vi "Athesim control.vi"() -> ()   [LabVIEW 2021]
uses:
  <vilib>/DAQmx/create/channels.llb/DAQmx Create Channel (DO-Digital Output).vi
  <vilib>/Instr/_visa.llb/VISA Configure Serial Port (Instr).vi
  <vilib>/DAQmx/write.llb/DAQmx Write (Analog DBL 1Chan 1Samp).vi
  <vilib>/DAQmx/write.llb/DAQmx Write (Digital Bool 1Line 1Point).vi
  <vilib>/DAQmx/read.llb/DAQmx Read (Digital Bool 1Line 1Point).vi
  <vilib>/measure/NI_MABase.lvlib
  <vilib>/DAQmx/create/channels.llb/DAQmx Create Channel (DI-Digital Input).vi
  <vilib>/DAQmx/write.llb/DAQmx Write (Analog Wfm 1Chan NSamp).vi
  <vilib>/DAQmx/create/channels.llb/DAQmx Create Channel (AO-Voltage-Basic).vi
panel:
  out "?":bool
  in  "Go live":bool
  in  "stop":bool=TRUE
  in  "Go SIM":bool
  in  "MG17Motor":refnum<k7>(container)
  in  "Tab Control":T1(tab)
  in  "acquire 405":bool
  in  "405 Exp":dbl=150.0
  out "Images needed":dbl=108.0
  in  "5 phases":bool
  in  "Exposure time":dbl=100.0
  in  "interval /s":dbl
  in  "Timepoints":u32=12 min=1 max=1000 step=1
  in  "647":bool
  in  "561":bool
  in  "488":bool
  in  "405":bool
  in  "Steps /um":dbl
  in  "z-slices":dbl=1.0
  in  "acquire 640":bool=TRUE
  in  "647 Exp":dbl=150.0
  in  "acquire 561":bool=TRUE
  in  "561 Exp":dbl=80.0
  in  "acquire 488":bool=TRUE
  in  "488 Exp":dbl=150.0
  in  "Live mode":T2(radio)=enum."Mirror 3"
  in  "Delay time":u32=50
  in  "Optosplit":T3(radio)=enum."rolling SIM"
  out "odd/even indicator":bool
  out "Current voltage":dbl=0.95 format="%#_13g"
  in  "Boolean":bool
  in  "Radio Buttons":enum32{"V1", "V2", "V3"}(radio)
  in  "Debug":dbl[](array[numeric])
  in  "647 voltages":dbl[][](array[numeric])=[[0.95, 2.25, 3.5], [0.950655, 2.25185, 3.50055], [0.95131, 2.2537, 3.5011]]
  in  "561 voltages":dbl[][](array[numeric])=[[0.95, 2.2, 3.45], [0.9508, 2.2025, 3.454], [0.9516, 2.205, 3.4548]]
  in  "488 voltages":dbl[][](array[numeric])=[[0.95, 2.25, 3.5], [0.950655, 2.25185, 3.50055], [0.95131, 2.2537, 3.5011]]
  in  "405 voltages":dbl[][](array[numeric])=[[1.0, 0.0, 0.0], [0.0, 0.0, 0.0], [0.0, 0.0, 4.0]]
  out "x+y":i32=4
  in  "647 voltages":dbl[][](array[numeric])=[[0.96, 2.2, 3.5], [0.97, 2.2035, 3.5085], [0.975, 2.2045, 3.5118]]
  in  "561 voltages":dbl[][](array[numeric])=[[0.85, 1.91, 3.2], [0.85065, 1.91064, 3.204], [0.85013, 1.91128, 3.208]]
  in  "488 voltages":dbl[][](array[numeric])=[[0.96, 2.2, 3.5], [0.97, 2.2045, 3.51], [0.975, 2.209, 3.52]]
  in  "405 voltages":dbl[][](array[numeric])=[[1.0, 0.0, 0.0], [0.0, 0.0, 0.0], [0.0, 0.0, 4.0]]
  in  "ASI stage channel":refnum<visa-resource-name>="COM5"
  in  "physical channels":tag="Dev1/ao0"
  in  "expose any":tag="Dev1/port0/line5"
  in  "647 Power":ext(slide)=34.85 scale=0.0..100.0
  in  "405 shutter":tag="Dev1/port0/line8"
  in  "561 shutter":tag="Dev1/port0/line0"
  in  "488 shutter":tag="Dev1/port0/line1"
  in  "Busy in":tag="Dev1/port0/line3"
  in  "Exposure out":tag="Dev1/port0/line2"
  in  "647 channel":refnum<visa-resource-name>="COM4"
  in  "561 power":dbl(slide)=0.15584415584415584 min=0.0 max=1.0 step=0.05 scale=0.0..1.0
  in  "Tab Control 2":T4(tab)
  out "Initialisation error":errorcluster
  out "stage error":errorcluster
  out "Camera/galvo error":errorcluster
  out "Laser error":errorcluster
  out "optosplit stage error":errorcluster
  out "resulting string":string="movrel z=0.000000 \r\n"
  out "resulting string 2":string="movrel z=-0.000000 \r\n"
  in  "short delay":dbl=5.0
  in  "long delay":dbl=55.0
  # "o"
  # "o"
  # "o"
  # "o"
  # "o"
  # "o"
  # "o"
  # "o"
  # "o"
  # "o"
  # "o"
  # "o"
  # "-60"
  # "0"
  # "60"
  # "-60"
  # "0"
  # "60"
  # "-60"
  # "0"
  # "60"
  # "-60"
  # "0"
  # "60"
  # "0"
  # "2p/3"
  # "4p/3"
  # "o"
  # "o"
  # "o"
  # "o"
  # "o"
  # "o"
  # "o"
  # "o"
  # "o"
  # "o"
  # "o"
  # "o"
  # "-60"
  # "0"
  # "60"
  # "-60"
  # "0"
  # "60"
  # "-60"
  # "0"
  # "60"
  # "-60"
  # "0"
  # "60"
  # "0"
  # "3p/5"
  # "5p/5"
  # "7p/5"
  # "9p/5"
  # "Camera lines"
  # "Laser control"
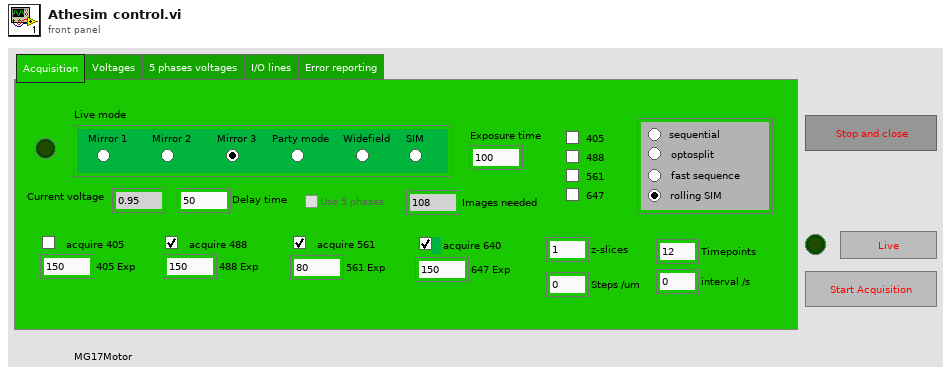
[diagram p1: front panel]
types:
  T1 = enum32{"Acquisition", "Voltages", "5 phases voltages", "I/O lines", "Error reporting"}
  T2 = enum32{"Mirror 1", "Mirror 2", "Mirror 3", "Party mode", "Widefield", "SIM"}
  T3 = enum32{"sequential", "optosplit", "fast sequence", "rolling SIM"}
  T4 = enum32{"Page 1", "Page 2", "Page 3", "Page 4", "Page 5"}
  T5 = enum8{"Enabled", "Disabled", "Disabled and Grayed Out"}
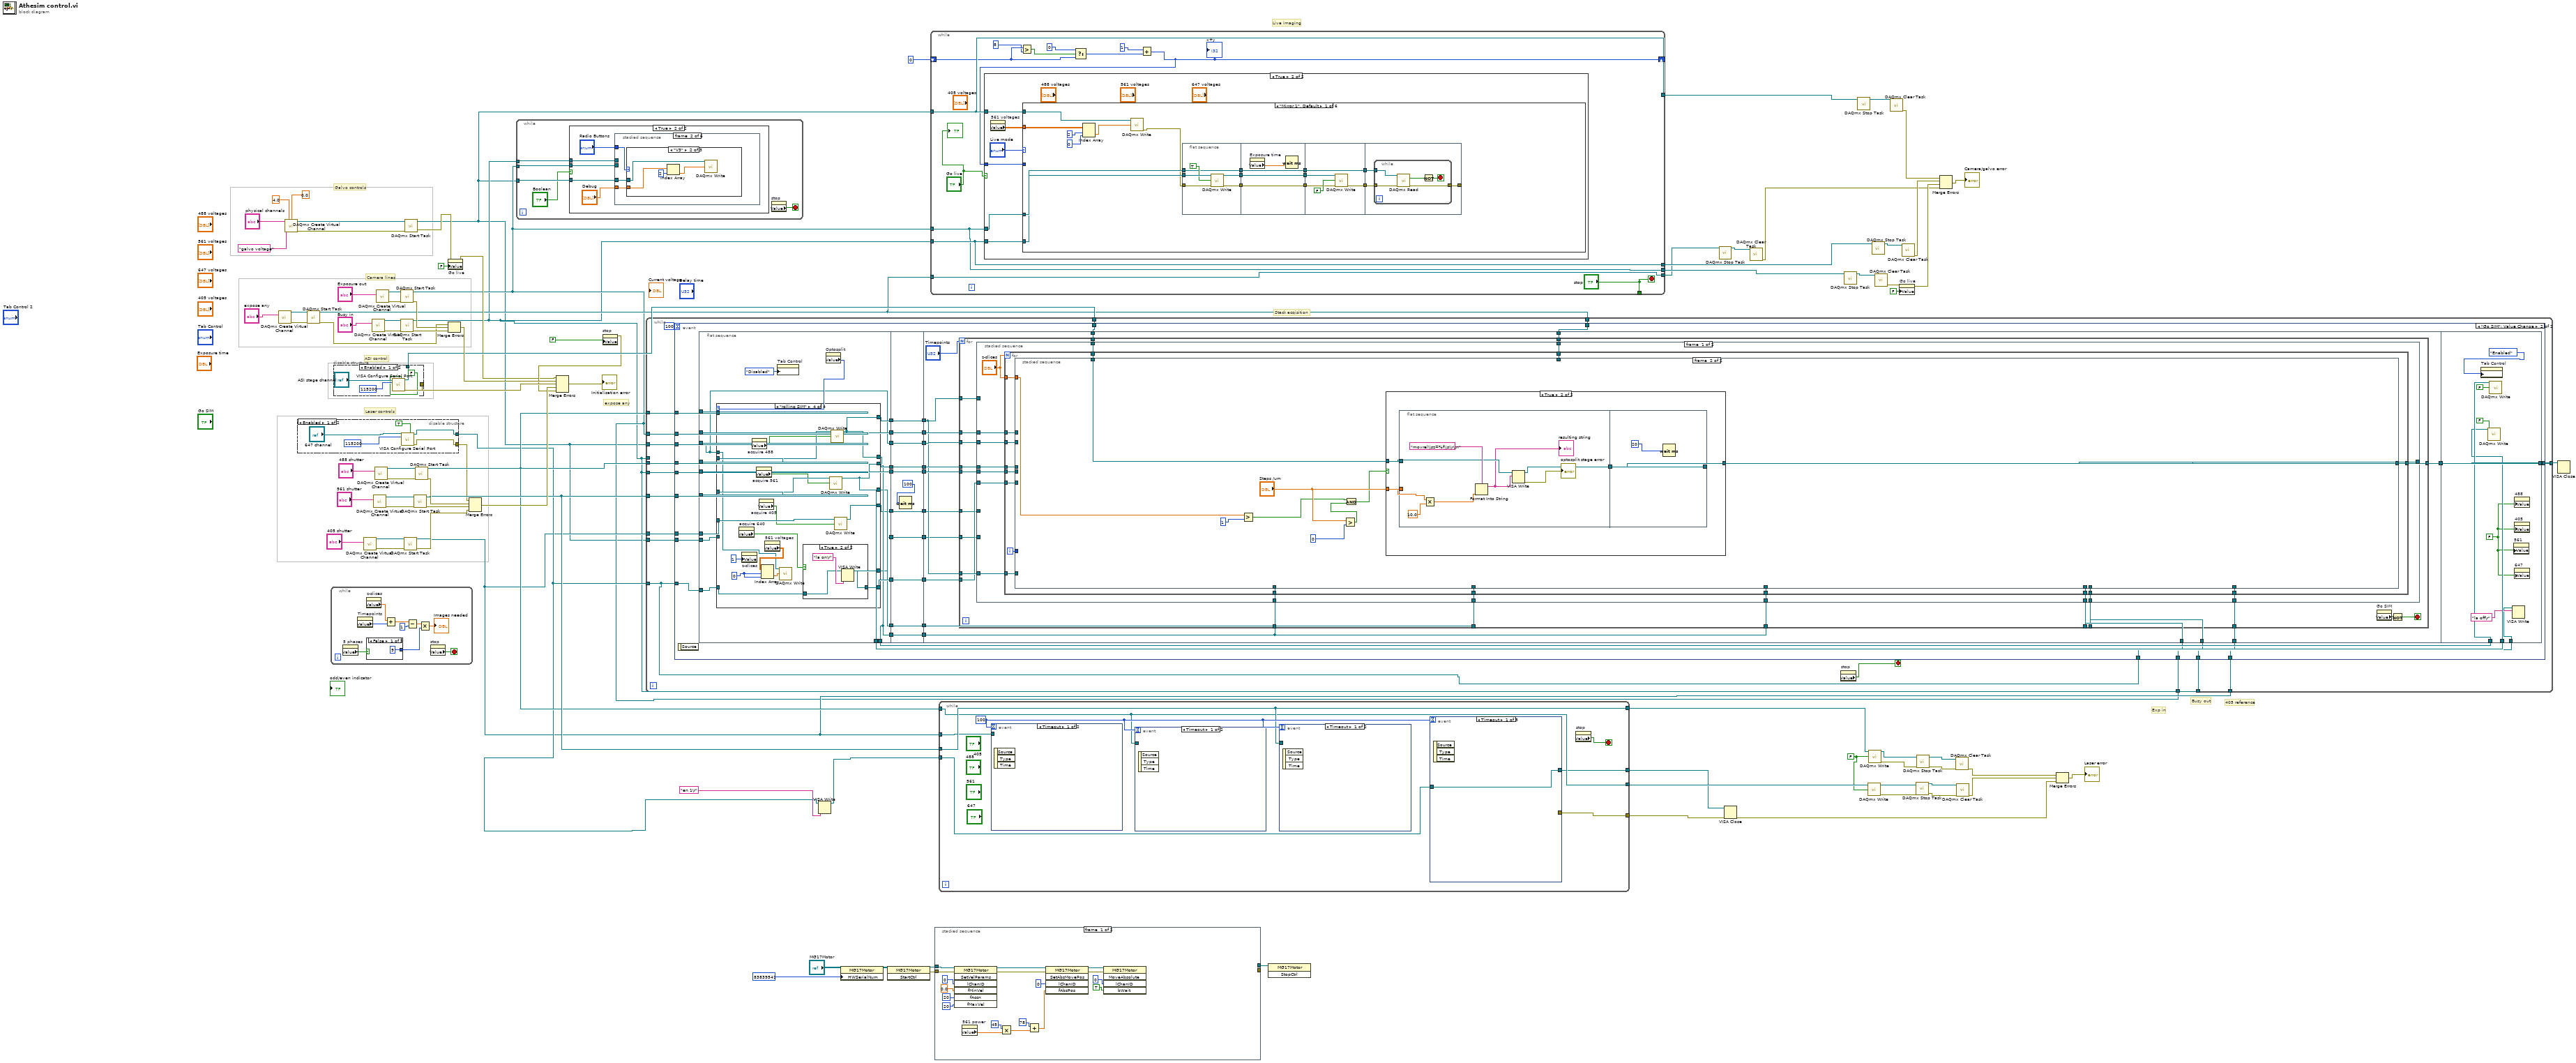
[diagram p0: block diagram]
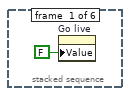
[diagram p3: hidden frame]
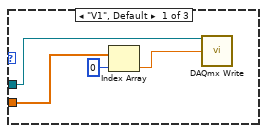
[diagram p4: hidden frame]
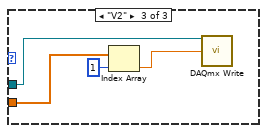
[diagram p5: hidden frame]
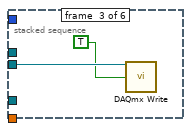
[diagram p6: hidden frame]
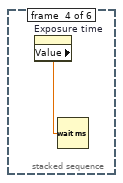
[diagram p7: hidden frame]
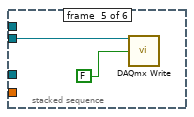
[diagram p8: hidden frame]
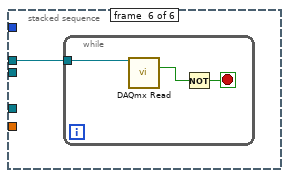
[diagram p9: hidden frame]
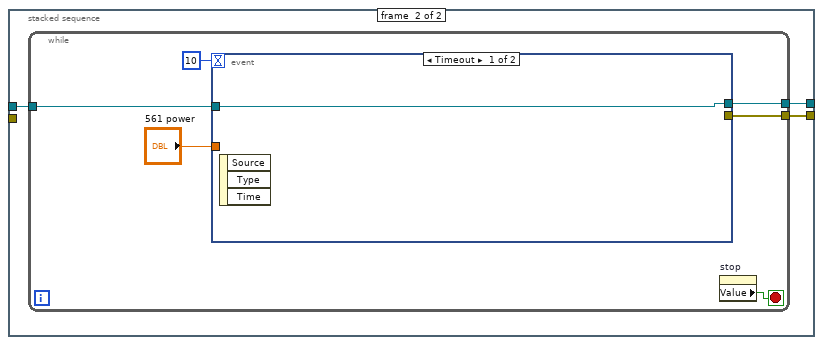
[diagram p10: hidden frame]
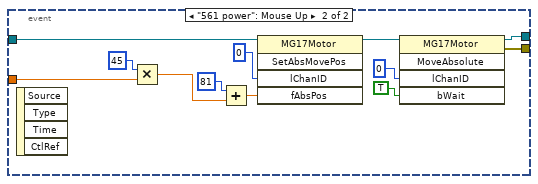
[diagram p11: hidden frame]
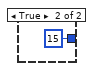
[diagram p13: hidden frame]
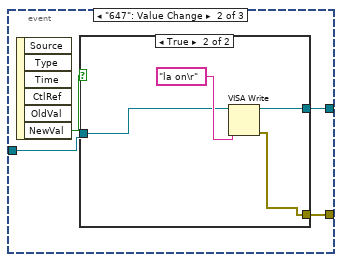
[diagram p15: hidden frame]
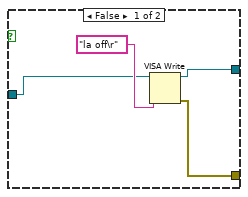
[diagram p16: hidden frame]
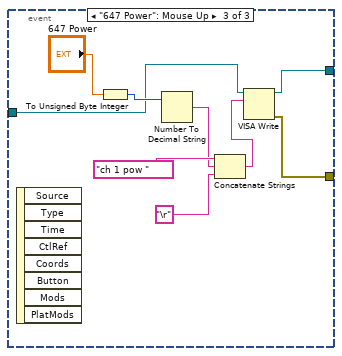
[diagram p17: hidden frame]
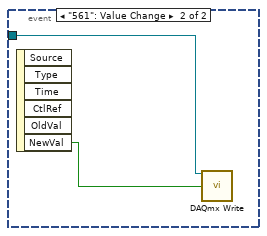
[diagram p18: hidden frame]
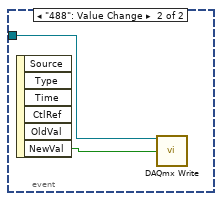
[diagram p19: hidden frame]
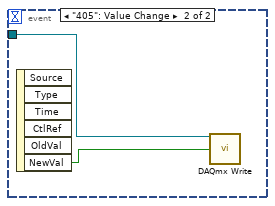
[diagram p20: hidden frame]
diagram:
  w58 = FALSE
  # "expose any"
  # "Busy out"
  # "Exp in"
  # "405 reference"
  # "Stack acqisition"
  # "Live imaging"
  # "Laser controls"
  # "ASI control"
  # "Camera lines"
  # "Galvo controls"
  n1 = call-poly <vilib>:"DAQmx Create Virtual Channel.vi"("lines"="expose any") -> ("task out"=w13:refnum<k21>, "error out"=w12:errorcluster)  [unwired: 13 in]
  n2 = call-poly <vilib>:"DAQmx Create Virtual Channel.vi"("maximum value"=4.0, "minimum value"=0.0, "physical channels"="physical channels", "name to assign"="galvo voltage") -> ("task out"=w6:refnum<k21>, "error out"=w5:errorcluster)  [unwired: 10 in]
  n3 = disable-structure shown="Enabled" {
    disable-tunnel: [w93 _] -> w27
    disable-tunnel: [w92 _] -> w29
    frame Enabled {
      n4 = call-poly "VISA Configure Serial Port"("VISA resource name"="647 channel", "Enable Termination\nChar (T)"=TRUE ("Enable Termination\nChar (T)"), "baud rate (9600)"=u32 115200) -> ("VISA resource name out"=w93:refnum<visa-resource-name>, "error out"=w92:errorcluster)  [unwired: 11 in]
    }
    frame Disabled {
    }
  }
  n5 = call <vilib>:"DAQmx Start Task.vi"("task/channels in"=w13, "error in"=w12) -> ("task out"=w10:refnum<k21>, "error out"=w11:errorcluster)  [unwired: 12 in]
  n6 = while {
    stop <- w97 stop-if-true
    n7 = property on="5 phases" class="Bool (strict)"() -> ("Value"=w105:bool)  [unwired: 2 in, 2 out]
    n8 = property on="Timepoints" class="DigNum (strict)"() -> ("Value"=w101:u32)  [unwired: 2 in, 2 out]
    n9 = property on="z-slices" class="DigNum (strict)"() -> ("Value"=w102:dbl)  [unwired: 2 in, 2 out]
    n10 = case shown="False" w105 {
      tunnel: [9 15] -> w104
      frame False {
      }
      frame True {
      }
    }
    n11 = Add(x=w102, y=w101) -> (x+y=w99:dbl)
    n12 = Subtract(x=w99, y=1) -> (x-y=w98:dbl)
    n13 = Multiply(x=w98, y=w104) -> (x*y=→"Images needed":dbl)
    n14 = property on="stop" class="Bool (strict)"() -> ("Value"=w97:bool)  [unwired: 2 in, 2 out]
  }
  n15 = disable-structure shown="Enabled" {
    disable-tunnel: [w110 _] -> w75
    disable-tunnel: [w109 _] -> w46
    frame Enabled {
      n16 = call-poly "VISA Configure Serial Port"("VISA resource name"="ASI stage channel", "Enable Termination\nChar (T)"=FALSE, "baud rate (9600)"=u32 115200) -> ("VISA resource name out"=w109:refnum<visa-resource-name>, "error out"=w110:errorcluster)  [unwired: 11 in]
    }
    frame Disabled {
    }
  }
  n17 = call-poly <vilib>:"DAQmx Create Virtual Channel.vi"("lines"="405 shutter") -> ("task out"=w40:refnum<k21>, "error out"=w41:errorcluster)  [unwired: 13 in]
  n18 = call-poly <vilib>:"DAQmx Create Virtual Channel.vi"("lines"="Busy in") -> ("task out"=w88:refnum<k21>, "error out"=w89:errorcluster)  [unwired: 13 in]
  n19 = call-poly <vilib>:"DAQmx Create Virtual Channel.vi"("lines"="561 shutter") -> ("task out"=w84:refnum<k21>, "error out"=w85:errorcluster)  [unwired: 13 in]
  n20 = call-poly <vilib>:"DAQmx Create Virtual Channel.vi"("lines"="488 shutter") -> ("task out"=w86:refnum<k21>, "error out"=w87:errorcluster)  [unwired: 13 in]
  n21 = call-poly <vilib>:"DAQmx Create Virtual Channel.vi"("lines"="Exposure out") -> ("task out"=w91:refnum<k21>, "error out"=w90:errorcluster)  [unwired: 13 in]
  n22 = call <vilib>:"DAQmx Start Task.vi"("task/channels in"=w91, "error in"=w90) -> ("task out"=w3:refnum<k21>, "error out"=w77:errorcluster)  [unwired: 12 in]
  n23 = call <vilib>:"DAQmx Start Task.vi"("task/channels in"=w88, "error in"=w89) -> ("task out"=w2:refnum<k21>, "error out"=w76:errorcluster)  [unwired: 12 in]
  n24 = call <vilib>:"DAQmx Start Task.vi"("task/channels in"=w40, "error in"=w41) -> ("task out"=w25:refnum<k21>, "error out"=w39:errorcluster)  [unwired: 12 in]
  n25 = call <vilib>:"DAQmx Start Task.vi"("task/channels in"=w6, "error in"=w5) -> ("task out"=w1:refnum<k21>, "error out"=w23:errorcluster)  [unwired: 12 in]
  n26 = call <vilib>:"DAQmx Start Task.vi"("task/channels in"=w84, "error in"=w85) -> ("task out"=w71:refnum<k21>, "error out"=w78:errorcluster)  [unwired: 12 in]
  n27 = call <vilib>:"DAQmx Start Task.vi"("task/channels in"=w86, "error in"=w87) -> ("task out"=w70:refnum<k21>, "error out"=w79:errorcluster)  [unwired: 12 in]
  n28 = property on="Go live" class="Bool (strict)"(error in=w23, "Value"=FALSE) -> (error out=w22:errorcluster)  [unwired: 1 in, 1 out]
  n29 = Merge Errors(w11, w77, w76) -> (w74:errorcluster)
  n30 = Merge Errors(w29, w79, w78, w39) -> (w73:errorcluster)
  n31 = while {
    tunnel: w3 -> [w116]
    tunnel: w2 -> [w115]
    tunnel: w1 -> [w114]
    stop <- w117 stop-if-true
    n32 = case shown="True" "Boolean" {
      tunnel: w116 -> [_ w122]
      tunnel: w115 -> [_ w121]
      tunnel: w114 -> [_ w120]
      frame False {
      }
      frame True {
        n33 = stacked-sequence {
          tunnel: w122 -> [_ _ w140 _ w142 _]
          tunnel: w121 -> [_ _ _ _ _ w145]
          tunnel: "Radio Buttons" -> [_ w126 _ _ _ _]
          tunnel: "Debug" -> [_ w125 _ _ _ _]
          tunnel: w120 -> [_ w124 _ _ _ _]
          frame #0 {
            n34 = property on="Go live" class="Bool (strict)"("Value"=FALSE ("Go live")) -> ()  [unwired: 2 in, 2 out]
          }
          frame #1 {
            n35 = case shown="\"V3\"" w126 {
              tunnel: w125 -> [w129 w133 w137]
              tunnel: w124 -> [w130 w134 w138]
              frame "V1", Default {
                n36 = Index Array(array=w129, index=0) -> (element=w128:dbl)
                n37 = call-poly <vilib>:"DAQmx Write.vi"("task/channels in"=w130, "data"=w128) -> ()  [unwired: 11 in, 3 out]
              }
              frame "V3" {
                n38 = Index Array(array=w133, index=2) -> (element=w132:dbl)
                n39 = call-poly <vilib>:"DAQmx Write.vi"("task/channels in"=w134, "data"=w132) -> ()  [unwired: 11 in, 3 out]
              }
              frame "V2" {
                n40 = Index Array(array=w137, index=1) -> (element=w136:dbl)
                n41 = call-poly <vilib>:"DAQmx Write.vi"("task/channels in"=w138, "data"=w136) -> ()  [unwired: 11 in, 3 out]
              }
            }
          }
          frame #2 {
            n42 = call-poly <vilib>:"DAQmx Write.vi"("task/channels in"=w140, "data"=TRUE) -> ()  [unwired: 11 in, 3 out]
          }
          frame #3 {
            n43 = property on="Exposure time" class="DigNum (strict)"() -> ("Value"=w141:dbl)  [unwired: 2 in, 2 out]
            n44 = Wait (ms)(milliseconds to wait=w141) -> ()  [unwired: 1 out]
          }
          frame #4 {
            n45 = call-poly <vilib>:"DAQmx Write.vi"("task/channels in"=w142, "data"=FALSE) -> ("error out"=w143:errorcluster)  [unwired: 11 in, 2 out]
          }
          frame #5 {
            n46 = while {
              tunnel: w145 -> [w146]
              stop <- w148 stop-if-true
              n47 = call-poly <vilib>:"DAQmx Read.vi"("task/channels in"=w146) -> ("data"=w147:bool)  [unwired: 12 in, 2 out]
              n48 = Not(x=w147) -> (.not. x?=w148:bool)
            }
          }
        }
      }
    }
    n49 = property on="stop" class="Bool (strict)"() -> ("Value"=w117:bool)  [unwired: 2 in, 2 out]
  }
  n50 = property on="stop" class="Bool (strict)"("Value"=FALSE) -> (error out=w43:errorcluster)  [unwired: 2 in, 1 out]
  n51 = Merge Errors(w22, w74, w75, w73, w43) -> (→"Initialisation error":errorcluster)
  n52 = while {
    tunnel: w3 -> [w164]
    tunnel: w2 -> [w163]
    tunnel: w1 -> [w162]
    tunnel: w70 -> [w161]
    tunnel: w71 -> [w160]
    tunnel: w70 -> [w159]
    tunnel: w46 -> [w157]
    tunnel: [w156] -> w45
    tunnel: w2 -> [_]
    tunnel: w27 -> [w154]
    tunnel: w25 -> [w155]
    tunnel: w25 -> [w153]
    tunnel: w3 -> [w152]
    tunnel: w2 -> [w151]
    tunnel: w1 -> [w150]
    tunnel: w10 -> [w149]
    stop <- w158 stop-if-true
    n53 = event shown="[1] \"Go SIM\": Value Change" {
      selector: _ -> [_ _]
      dyn-events: _ -> [_ _]
      timeout: 100 -> [_ _]
      tunnel: w164 -> [_ w205]
      tunnel: w163 -> [_ w204]
      tunnel: w162 -> [_ w203]
      tunnel: w161 -> [_ w202]
      tunnel: w160 -> [_ w201]
      tunnel: w159 -> [_ w200]
      tunnel: w157 -> [w166 w199]
      tunnel: [w166 w198] -> w156
      tunnel: w154 -> [_ w194]
      tunnel: w155 -> [_ w193]
      tunnel: w154 -> [_ w192]
      tunnel: w153 -> [_ w191]
      tunnel: w152 -> [_ w190]
      tunnel: w151 -> [_ w189]
      tunnel: w150 -> [_ w188]
      tunnel: w149 -> [_ w167]
      event Timeout {
        n54 = event-data() -> ()  [unwired: 1 in, 3 out]
      }
      event "Go SIM": Value Change {
        n55 = event-data() -> ()  [unwired: 1 in, 1 out]
        n56 = flat-sequence {
          tunnel: [w223] -> w187
          tunnel: w205 -> [w223]
          tunnel: [w222] -> w185
          tunnel: w204 -> [w222]
          tunnel: [w207] -> w183
          tunnel: w203 -> [w207]
          tunnel: w202 -> [w220]
          tunnel: w201 -> [w219]
          tunnel: w200 -> [w218]
          tunnel: [w217] -> w181
          tunnel: [w216] -> w179
          tunnel: [w212] -> w195
          tunnel: [w211] -> w196
          tunnel: w194 -> [w215]
          tunnel: w193 -> [w214]
          tunnel: [w213] -> w177
          tunnel: [w212] -> w175
          tunnel: [w211] -> w173
          tunnel: w188 -> [w210]
          tunnel: [w209] -> w170
          tunnel: [w208] -> w168
          tunnel: w187 -> [w313]
          tunnel: [w313] -> w186
          tunnel: w185 -> [w312]
          tunnel: [w312] -> w184
          tunnel: w183 -> [w311]
          tunnel: [w311] -> w182
          tunnel: w181 -> [w310]
          tunnel: [w310] -> w180
          tunnel: w179 -> [w309]
          tunnel: [w309] -> w178
          tunnel: w177 -> [w308]
          tunnel: [w308] -> w176
          tunnel: w175 -> [w307]
          tunnel: [w307] -> w174
          tunnel: w173 -> [w306]
          tunnel: [w306] -> w172
          tunnel: [w304] -> w171
          tunnel: w170 -> [w304]
          tunnel: [w303] -> w169
          tunnel: w168 -> [w303]
          tunnel: w186 -> [w329]
          tunnel: w184 -> [w328]
          tunnel: w182 -> [w327]
          tunnel: w180 -> [w326]
          tunnel: w178 -> [w317]
          tunnel: w199 -> [w325]
          tunnel: [w324] -> w197
          tunnel: w176 -> [w323]
          tunnel: w174 -> [w321]
          tunnel: w172 -> [w322]
          tunnel: w191 -> [w320]
          tunnel: w190 -> [w319]
          tunnel: w189 -> [w318]
          tunnel: w171 -> [w316]
          tunnel: w169 -> [w315]
          tunnel: w167 -> [w314]
          tunnel: [w1125] -> w198
          tunnel: w197 -> [w1125]
          tunnel: w196 -> [w1121]
          tunnel: w195 -> [w1122]
          tunnel: w192 -> [w1119]
          frame #0 {
            n57 = property on="Tab Control" class="TabCtl (strict)"("DisabledEnum"=T5."Disabled" ("Disabled")) -> ()  [unwired: 2 in, 2 out]
            n58 = property on="Optosplit" class="RadioBtnsControl (strict)"() -> ("Value"=w221:T3)  [unwired: 2 in, 2 out]
            n59 = case shown="\"rolling SIM\"" w221 {
              tunnel: w220 -> [_ _ _ _]
              tunnel: w219 -> [w234 w256 w275 w294]
              tunnel: w218 -> [w235 w257 w277 w296]
              tunnel: [w233 w255 w274 w293] -> w217
              tunnel: [w232 w254 w276 w295] -> w216
              tunnel: [w233 w255 w274 w293] -> w211
              tunnel: [w232 w254 w276 w295] -> w212
              tunnel: w215 -> [w227 w249 w272 w292]
              tunnel: w214 -> [w230 w252 w270 w291]
              tunnel: [w224 w246 w268 w289] -> w213
              tunnel: [w228 w250 w269 w290] -> w209
              tunnel: w210 -> [w225 w248 _ _]
              tunnel: [w224 w246 w268 w289] -> w208
              tunnel: w207 -> [_ _ _ w280]
              frame "sequential", Default {
                n60 = property on="odd/even indicator" class="Bool (strict)"() -> ("Value"=w226:bool)  [unwired: 2 in, 2 out]
                n61 = case shown="True" w226 {
                  tunnel: w225 -> [w241 w245]
                  frame False {
                    w239 = 2
                    n62 = property on="647 voltages" class="Arr (strict)"() -> ("Value"=w240:dbl[][])  [unwired: 2 in, 2 out]
                    n63 = Index Array(array=w240, index (row)=w239, index (col)=w239) -> (element=w238:dbl)
                    n64 = call-poly <vilib>:"DAQmx Write.vi"("task/channels in"=w241, "data"=w238) -> ()  [unwired: 11 in, 3 out]
                  }
                  frame True {
                    w243 = 0
                    n65 = property on="561 voltages" class="Arr (strict)"() -> ("Value"=w244:dbl[][])  [unwired: 2 in, 2 out]
                    n66 = Index Array(array=w244, index (row)=w243, index (col)=w243) -> (element=w242:dbl)
                    n67 = call-poly <vilib>:"DAQmx Write.vi"("task/channels in"=w245, "data"=w242) -> ()  [unwired: 11 in, 3 out]
                  }
                }
                n68 = call-poly <vilib>:"DAQmx Write.vi"("task/channels in"=w230, "data"=FALSE) -> ("task out"=w228:refnum<k21>)  [unwired: 11 in, 2 out]
                n69 = call-poly <vilib>:"DAQmx Write.vi"("task/channels in"=w234, "data"=FALSE) -> ("task out"=w233:refnum<k21>)  [unwired: 11 in, 2 out]
                n70 = call-poly <vilib>:"DAQmx Write.vi"("task/channels in"=w235, "data"=FALSE) -> ("task out"=w232:refnum<k21>)  [unwired: 11 in, 2 out]
                n71 = VISA Write(VISA resource name=w227, write buffer="la off\r" ("format string")) -> (VISA resource name out=w224:refnum<visa-resource-name>)  [unwired: 1 in, 2 out]
              }
              frame "fast sequence" {
                n72 = property on="odd/even indicator" class="Bool (strict)"() -> ("Value"=w247:bool)  [unwired: 2 in, 2 out]
                n73 = case shown="True" w247 {
                  tunnel: w248 -> [w263 w267]
                  frame False {
                    w261 = 2
                    n74 = property on="647 voltages" class="Arr (strict)"() -> ("Value"=w262:dbl[][])  [unwired: 2 in, 2 out]
                    n75 = Index Array(array=w262, index (row)=w261, index (col)=w261) -> (element=w260:dbl)
                    n76 = call-poly <vilib>:"DAQmx Write.vi"("task/channels in"=w263, "data"=w260) -> ()  [unwired: 11 in, 3 out]
                  }
                  frame True {
                    w265 = 0
                    n77 = property on="647 voltages" class="Arr (strict)"() -> ("Value"=w266:dbl[][])  [unwired: 2 in, 2 out]
                    n78 = Index Array(array=w266, index (row)=w265, index (col)=w265) -> (element=w264:dbl)
                    n79 = call-poly <vilib>:"DAQmx Write.vi"("task/channels in"=w267, "data"=w264) -> ()  [unwired: 11 in, 3 out]
                  }
                }
                n80 = call-poly <vilib>:"DAQmx Write.vi"("task/channels in"=w252, "data"=FALSE) -> ("task out"=w250:refnum<k21>)  [unwired: 11 in, 2 out]
                n81 = call-poly <vilib>:"DAQmx Write.vi"("task/channels in"=w256, "data"=FALSE) -> ("task out"=w255:refnum<k21>)  [unwired: 11 in, 2 out]
                n82 = call-poly <vilib>:"DAQmx Write.vi"("task/channels in"=w257, "data"=FALSE) -> ("task out"=w254:refnum<k21>)  [unwired: 11 in, 2 out]
                n83 = VISA Write(VISA resource name=w249, write buffer="la off\r" ("format string")) -> (VISA resource name out=w246:refnum<visa-resource-name>)  [unwired: 1 in, 2 out]
              }
              frame "optosplit" {
                n84 = call-poly <vilib>:"DAQmx Write.vi"("task/channels in"=w275, "data"=TRUE) -> ("task out"=w274:refnum<k21>)  [unwired: 11 in, 2 out]
                n85 = call-poly <vilib>:"DAQmx Write.vi"("task/channels in"=w277, "data"=TRUE) -> ("task out"=w276:refnum<k21>)  [unwired: 11 in, 2 out]
                n86 = call-poly <vilib>:"DAQmx Write.vi"("task/channels in"=w270, "data"=TRUE) -> ("task out"=w269:refnum<k21>)  [unwired: 11 in, 2 out]
                n87 = VISA Write(VISA resource name=w272, write buffer="la on\r" ("format string")) -> (VISA resource name out=w268:refnum<visa-resource-name>)  [unwired: 1 in, 2 out]
              }
              frame "rolling SIM" {
                w285 = 0
                n88 = property on="acquire 640" class="Bool (strict)"() -> ("Value"=w281:bool)  [unwired: 2 in, 2 out]
                n89 = property on="z-slices" class="DigNum (strict)"("Value"=1) -> ()  [unwired: 2 in, 2 out]
                n90 = property on="acquire 488" class="Bool (strict)"() -> ("Value"=w284:bool)  [unwired: 2 in, 2 out]
                n91 = property on="acquire 561" class="Bool (strict)"() -> ("Value"=w283:bool)  [unwired: 2 in, 2 out]
                n92 = property on="acquire 405" class="Bool (strict)"() -> ("Value"=w282:bool)  [unwired: 2 in, 2 out]
                n93 = property on="561 voltages" class="Arr (strict)"() -> ("Value"=w286:dbl[][])  [unwired: 2 in, 2 out]
                n94 = Index Array(array=w286, index (row)=w285, index (col)=w285) -> (element=w287:dbl)
                n95 = call-poly <vilib>:"DAQmx Write.vi"("task/channels in"=w280, "data"=w287) -> ()  [unwired: 11 in, 3 out]
                n96 = case shown="True" w281 {
                  tunnel: w292 -> [w298 w301]
                  tunnel: [w297 w300] -> w289
                  frame False {
                    n97 = VISA Write(VISA resource name=w298, write buffer="la off\r" ("format string")) -> (VISA resource name out=w297:refnum<visa-resource-name>)  [unwired: 1 in, 2 out]
                  }
                  frame True {
                    n98 = VISA Write(VISA resource name=w301, write buffer="la on\r" ("format string")) -> (VISA resource name out=w300:refnum<visa-resource-name>)  [unwired: 1 in, 2 out]
                  }
                }
                n99 = call-poly <vilib>:"DAQmx Write.vi"("task/channels in"=w294, "data"=w283) -> ("task out"=w293:refnum<k21>)  [unwired: 11 in, 2 out]
                n100 = call-poly <vilib>:"DAQmx Write.vi"("task/channels in"=w296, "data"=w284) -> ("task out"=w295:refnum<k21>)  [unwired: 11 in, 2 out]
                n101 = call-poly <vilib>:"DAQmx Write.vi"("task/channels in"=w291, "data"=w282) -> ("task out"=w290:refnum<k21>)  [unwired: 11 in, 2 out]
              }
            }
          }
          frame #1 {
            n102 = Wait (ms)(milliseconds to wait=100) -> ()  [unwired: 1 out]
          }
          frame #2 {
            n103 = for {
              N: "Timepoints" -> [_]
              tunnel: w329 -> [w350]
              tunnel: w328 -> [w349]
              tunnel: w327 -> [w348]
              tunnel: w326 -> [w347]
              tunnel: w317 -> [w346]
              tunnel: w325 -> [w345]
              tunnel: [w344] -> w324
              tunnel: w323 -> [w343]
              tunnel: w322 -> [w342]
              tunnel: w321 -> [w341]
              tunnel: w321 -> [w340]
              tunnel: w320 -> [w339]
              tunnel: w319 -> [w338]
              tunnel: w318 -> [w337]
              tunnel: w317 -> [w336]
              tunnel: w316 -> [w335]
              tunnel: w315 -> [w334]
              tunnel: w314 -> [w333]
              stop <- w331 stop-if-true
              n104 = stacked-sequence {
                tunnel: w350 -> [w366 _]
                tunnel: w349 -> [w365 _]
                tunnel: w348 -> [w364 _]
                tunnel: w347 -> [w363 w1030]
                tunnel: w346 -> [w362 _]
                tunnel: w345 -> [w361 w1032]
                tunnel: [w360 _] -> w344
                tunnel: w343 -> [w359 _]
                tunnel: w342 -> [w358 _]
                tunnel: w341 -> [w357 _]
                tunnel: w340 -> [w356 _]
                tunnel: w339 -> [w355 _]
                tunnel: w338 -> [w354 _]
                tunnel: w337 -> [w353 _]
                tunnel: w336 -> [_ w1031]
                tunnel: w335 -> [_ w1029]
                tunnel: w334 -> [_ w1028]
                tunnel: w333 -> [w351 _]
                frame #0 {
                  n105 = for {
                    N: "z-slices" -> [_]
                    tunnel: w366 -> [w383]
                    tunnel: w365 -> [w382]
                    tunnel: w364 -> [w381]
                    tunnel: w363 -> [w380]
                    tunnel: w362 -> [w379]
                    tunnel: w361 -> [w378]
                    tunnel: [w377] -> w360
                    tunnel: w359 -> [w376]
                    tunnel: w358 -> [w375]
                    tunnel: w357 -> [w374]
                    tunnel: w356 -> [w373]
                    tunnel: w355 -> [w372]
                    tunnel: w354 -> [w371]
                    tunnel: w353 -> [w370]
                    tunnel: "z-slices" -> [w368]
                    tunnel: w351 -> [w367]
                    i -> [w369]
                    n106 = stacked-sequence {
                      tunnel: w383 -> [w398 _]
                      tunnel: w382 -> [w397 _]
                      tunnel: w381 -> [w396 _]
                      tunnel: w380 -> [w395 _]
                      tunnel: w379 -> [w394 _]
                      tunnel: w378 -> [_ w1000]
                      tunnel: [_ w999] -> w377
                      tunnel: w376 -> [w392 _]
                      tunnel: w375 -> [w391 _]
                      tunnel: w374 -> [w390 _]
                      tunnel: w373 -> [w389 _]
                      tunnel: w372 -> [w388 _]
                      tunnel: w371 -> [w387 _]
                      tunnel: w370 -> [w386 _]
                      tunnel: w369 -> [w385 _]
                      tunnel: w368 -> [_ w995]
                      tunnel: w367 -> [w384 _]
                      frame #0 {
                        n107 = case shown="\"rolling SIM\"" "Optosplit" {
                          tunnel: w398 -> [w421 w744 w873 w970]
                          tunnel: w397 -> [w420 w743 w872 w969]
                          tunnel: w396 -> [w403 w739 w871 w963]
                          tunnel: w395 -> [w410 _ _ _]
                          tunnel: w394 -> [w409 _ _ _]
                          tunnel: "5 phases" -> [_ _ w870 _]
                          tunnel: w392 -> [w408 w738 _ _]
                          tunnel: w391 -> [w407 w737 _ _]
                          tunnel: w390 -> [w406 _ _ _]
                          tunnel: w389 -> [_ w732 _ _]
                          tunnel: w388 -> [w405 w731 _ _]
                          tunnel: w387 -> [w402 _ _ _]
                          tunnel: w386 -> [w401 _ _ _]
                          tunnel: w385 -> [_ _ _ _]
                          tunnel: w384 -> [w400 w730 w869 w964]
                          frame "sequential", Default {
                            # "Without optosplit"
                            n108 = case shown="True" "acquire 640" {
                              tunnel: w421 -> [w649 w659]
                              tunnel: w420 -> [w647 w658]
                              tunnel: w403 -> [w648 w652]
                              tunnel: [w649 w656] -> w416
                              tunnel: [w648 w657] -> w417
                              tunnel: [w647 w655] -> w418
                              tunnel: w408 -> [_ w651]
                              tunnel: w400 -> [_ w650]
                              frame False {
                              }
                              frame True {
                                n109 = property on="647 voltages" class="Arr (strict)"() -> ("Value"=w653:dbl[][])  [unwired: 2 in, 2 out]
                                n110 = stacked-sequence {
                                seq-local: [_ w673 _ _] -> [_ _ w693 _]
                                seq-local: [_ w672 _ _] -> [_ _ w692 _]
                                seq-local: [_ w671 _ _] -> [_ _ w691 _]
                                seq-local: [_ w670 _ _] -> [_ _ w687 _]
                                seq-local: [_ w669 _ _] -> [_ _ w686 _]
                                tunnel: w659 -> [_ w673 _ _]
                                tunnel: w652 -> [_ w672 _ _]
                                tunnel: w658 -> [_ w671 _ _]
                                tunnel: w653 -> [_ w670 _ _]
                                tunnel: "647 Exp" -> [_ w669 _ _]
                                tunnel: [_ _ w690 _] -> w657
                                tunnel: [_ _ w689 _] -> w656
                                tunnel: [_ _ w688 _] -> w655
                                tunnel: w653 -> [_ w668 _ _]
                                tunnel: w652 -> [_ w667 _ _]
                                tunnel: w651 -> [w660 _ _ w727]
                                tunnel: w650 -> [_ _ w684 _]
                                frame #0 {
                                n111 = stacked-sequence {
                                tunnel: w660 -> [w661 _]
                                frame #0 {
                                n112 = VISA Write(VISA resource name=w661, write buffer="la on\r" ("format string")) -> ()  [unwired: 1 in, 3 out]
                                }
                                frame #1 {
                                n113 = Wait (ms)(milliseconds to wait=100) -> ()  [unwired: 1 out]
                                }
                                }
                                }
                                frame #1 {
                                n114 = property on="odd/even indicator" class="Bool (strict)"() -> ("Value"=w664:bool)  [unwired: 2 in, 2 out]
                                n115 = case shown="False" w664 {
                                tunnel: [2 0] -> w666
                                tunnel: [2 0] -> w665
                                frame False {
                                }
                                frame True {
                                }
                                }
                                n116 = flat-sequence {
                                tunnel: [w681] -> _
                                tunnel: w668 -> [w683]
                                tunnel: w667 -> [w681]
                                tunnel: [w682] -> _
                                tunnel: w666 -> [w679]
                                tunnel: w665 -> [w678]
                                frame #0 {
                                n117 = Index Array(array=w683, index (row)=w679, index (col)=w678) -> (element=w680:dbl)
                                n118 = call-poly <vilib>:"DAQmx Write.vi"("task/channels in"=w681, "data"=w680) -> ("task out"=w682:refnum<k21>)  [unwired: 11 in, 2 out]
                                }
                                }
                                }
                                frame #2 {
                                n119 = for {
                                N: 9 -> [_]
                                tunnel: w687 -> [w705]
                                tunnel: w693 -> [w702]
                                tunnel: w692 -> [w703]
                                tunnel: w691 -> [w701]
                                tunnel: w686 -> [w704]
                                tunnel: [w703] -> w690
                                tunnel: [w702] -> w689
                                tunnel: [w701] -> w688
                                tunnel: w684 -> [w694]
                                i -> [w697]
                                n120 = property on="odd/even indicator" class="Bool (strict)"() -> ("Value"=w695:bool)  [unwired: 2 in, 2 out]
                                n121 = case shown="True" w695 {
                                tunnel: [i32[] [1, 0, 2, 1, 0, 2, 1, 0, 0, 0, 1, 2, 3, 4, 0] i32[] [1, 2, 0, 1, 2, 0, 1, 2, 2, 0, 1, 2, 3, 4, 0]] -> w700
                                tunnel: [i32[] [2, 2, 1, 1, 1, 0, 0, 0, 0, 2, 2, 2, 2, 2, 0] i32[] [0, 0, 1, 1, 1, 2, 2, 2, 2, 2, 2, 2, 2, 2, 0]] -> w699
                                frame False {
                                }
                                frame True {
                                }
                                }
                                n122 = Index Array(array=w700, index=w697) -> (element=w698:i32)
                                n123 = flat-sequence {
                                tunnel: w705 -> [w714]
                                tunnel: w704 -> [w718]
                                tunnel: w703 -> [w717]
                                tunnel: w702 -> [w716]
                                tunnel: w701 -> [w715]
                                tunnel: w696 -> [w712]
                                tunnel: w698 -> [w711]
                                tunnel: w694 -> [w710]
                                frame #0 {
                                n124 = Index Array(array=w714, index (row)=w711, index (col)=w712) -> (element=w713:dbl)
                                n125 = call "take image.vi"("Voltage"=w713, "Exposure time"=w718, "expose any"=w710, "Busy out"=w715, "Exp In"=w716, "Galvo"=w717) -> ()  [unwired: 6 in]
                                }
                                frame #1 {
                                n126 = property on="Delay time" class="DigNum (strict)"() -> ("Value"=w719:u32)  [unwired: 2 in, 2 out]
                                n127 = Wait (ms)(milliseconds to wait=w719) -> ()  [unwired: 1 out]
                                }
                                }
                                n128 = Index Array(array=w699, index=w697) -> (element=w696:i32)
                                }
                                }
                                frame #3 {
                                n129 = property on="acquire 488" class="Bool (strict)"() -> ("Value"=w723:bool)  [unwired: 2 in, 2 out]
                                n130 = property on="acquire 405" class="Bool (strict)"() -> ("Value"=w722:bool)  [unwired: 2 in, 2 out]
                                n131 = property on="acquire 561" class="Bool (strict)"() -> ("Value"=w724:bool)  [unwired: 2 in, 2 out]
                                n132 = property on="odd/even indicator" class="Bool (strict)"() -> ("Value"=w725:bool)  [unwired: 2 in, 2 out]
                                n133 = Or(x=w724, y=w723) -> (x .or. y?=w721:bool)
                                n134 = Not(x=w725) -> (.not. x?=w726:bool)
                                n135 = Or(x=w721, y=w722) -> (x .or. y?=w720:bool)
                                n136 = case shown="True" w720 {
                                tunnel: w727 -> [_ w728]
                                frame False {
                                }
                                frame True {
                                n137 = VISA Write(VISA resource name=w728, write buffer="la off\r" ("format string")) -> ()  [unwired: 1 in, 3 out]
                                }
                                }
                                n138 = property on="odd/even indicator" class="Bool (strict)"("Value"=w726) -> ()  [unwired: 2 in, 2 out]
                                }
                                }
                              }
                            }
                            n139 = case shown="True" "acquire 561" {
                              tunnel: w418 -> [w566 w577]
                              tunnel: w417 -> [w567 w578]
                              tunnel: [w565 w575] -> w414
                              tunnel: [w567 w576] -> w413
                              tunnel: [w566 w574] -> w412
                              tunnel: w416 -> [w565 w573]
                              tunnel: w410 -> [_ _]
                              tunnel: w403 -> [_ w570]
                              tunnel: w407 -> [_ w569]
                              tunnel: w400 -> [_ w568]
                              frame False {
                              }
                              frame True {
                                n140 = property on="561 voltages" class="Arr (strict)"() -> ("Value"=w571:dbl[][])  [unwired: 2 in, 2 out]
                                n141 = stacked-sequence {
                                seq-local: [_ w588 _ _] -> [_ _ w610 _]
                                seq-local: [_ w587 _ _] -> [_ _ w609 _]
                                seq-local: [_ w586 _ _] -> [_ _ w605 _]
                                seq-local: [_ w585 _ _] -> [_ _ w603 _]
                                seq-local: [_ w584 _ _] -> [_ _ w602 _]
                                tunnel: w578 -> [_ w588 _ _]
                                tunnel: w577 -> [_ w587 _ _]
                                tunnel: w573 -> [_ w586 _ _]
                                tunnel: w571 -> [_ w585 _ _]
                                tunnel: "561 Exp" -> [_ w584 _ _]
                                tunnel: [_ _ w608 _] -> w576
                                tunnel: [_ _ w607 _] -> w575
                                tunnel: [_ _ w606 _] -> w574
                                tunnel: w571 -> [_ w582 _ _]
                                tunnel: w570 -> [_ w581 _ _]
                                tunnel: w569 -> [w580 _ _ w644]
                                tunnel: w568 -> [_ _ w601 _]
                                frame #0 {
                                n142 = call-poly <vilib>:"DAQmx Write.vi"("task/channels in"=w580, "data"=TRUE) -> ()  [unwired: 11 in, 3 out]
                                }
                                frame #1 {
                                n143 = flat-sequence {
                                tunnel: w582 -> [w592]
                                tunnel: [w591] -> w583
                                tunnel: w581 -> [w590]
                                tunnel: [w600] -> _
                                tunnel: w583 -> [w600]
                                frame #0 {
                                n144 = property on="odd/even indicator" class="Bool (strict)"() -> ("Value"=w589:bool)  [unwired: 2 in, 2 out]
                                n145 = case shown="True" w589 {
                                tunnel: [2 0] -> w595
                                tunnel: [2 0] -> w594
                                frame False {
                                }
                                frame True {
                                }
                                }
                                n146 = Index Array(array=w592, index (row)=w595, index (col)=w594) -> (element=w593:dbl)
                                n147 = call-poly <vilib>:"DAQmx Write.vi"("task/channels in"=w590, "data"=w593) -> ("task out"=w591:refnum<k21>)  [unwired: 11 in, 2 out]
                                }
                                frame #1 {
                                }
                                }
                                }
                                frame #2 {
                                n148 = for {
                                N: 9 -> [_]
                                tunnel: w603 -> [w622]
                                tunnel: w605 -> [w619]
                                tunnel: w610 -> [w620]
                                tunnel: w609 -> [w618]
                                tunnel: w602 -> [w621]
                                tunnel: [w620] -> w608
                                tunnel: [w619] -> w607
                                tunnel: [w618] -> w606
                                tunnel: w601 -> [w611]
                                i -> [w615]
                                n149 = property on="odd/even indicator" class="Bool (strict)"() -> ("Value"=w612:bool)  [unwired: 2 in, 2 out]
                                n150 = case shown="False" w612 {
                                tunnel: [i32[] [2, 2, 1, 1, 1, 0, 0, 0, 0, 2, 2, 2, 2, 2, 0] i32[] [0, 0, 1, 1, 1, 2, 2, 2, 2, 2, 2, 2, 2, 2, 0]] -> w617
                                tunnel: [i32[] [1, 0, 2, 1, 0, 2, 1, 0, 0, 0, 1, 2, 3, 4, 0] i32[] [1, 2, 0, 1, 2, 0, 1, 2, 2, 0, 1, 2, 3, 4, 0]] -> w616
                                frame False {
                                }
                                frame True {
                                }
                                }
                                n151 = flat-sequence {
                                tunnel: w622 -> [w631]
                                tunnel: w621 -> [w635]
                                tunnel: w620 -> [w634]
                                tunnel: w619 -> [w633]
                                tunnel: w618 -> [w632]
                                tunnel: w614 -> [w629]
                                tunnel: w613 -> [w628]
                                tunnel: w611 -> [w627]
                                frame #0 {
                                n152 = Index Array(array=w631, index (row)=w629, index (col)=w628) -> (element=w630:dbl)
                                n153 = call "take image.vi"("Voltage"=w630, "Exposure time"=w635, "expose any"=w627, "Busy out"=w632, "Exp In"=w633, "Galvo"=w634) -> ()  [unwired: 6 in]
                                }
                                frame #1 {
                                n154 = property on="Delay time" class="DigNum (strict)"() -> ("Value"=w636:u32)  [unwired: 2 in, 2 out]
                                n155 = Wait (ms)(milliseconds to wait=w636) -> ()  [unwired: 1 out]
                                }
                                }
                                n156 = Index Array(array=w616, index=w615) -> (element=w614:i32)
                                n157 = Index Array(array=w617, index=w615) -> (element=w613:i32)
                                }
                                }
                                frame #3 {
                                n158 = property on="acquire 488" class="Bool (strict)"() -> ("Value"=w640:bool)  [unwired: 2 in, 2 out]
                                n159 = property on="acquire 405" class="Bool (strict)"() -> ("Value"=w641:bool)  [unwired: 2 in, 2 out]
                                n160 = property on="acquire 640" class="Bool (strict)"() -> ("Value"=w639:bool)  [unwired: 2 in, 2 out]
                                n161 = Or(x=w640, y=w641) -> (x .or. y?=w638:bool)
                                n162 = Or(x=w638, y=w639) -> (x .or. y?=w637:bool)
                                n163 = case shown="False" w637 {
                                tunnel: w644 -> [_ w645]
                                frame False {
                                }
                                frame True {
                                n164 = call-poly <vilib>:"DAQmx Write.vi"("task/channels in"=w645, "data"=FALSE) -> ()  [unwired: 11 in, 3 out]
                                }
                                }
                                n165 = property on="odd/even indicator" class="Bool (strict)"() -> ("Value"=w643:bool)  [unwired: 2 in, 2 out]
                                n166 = Not(x=w643) -> (.not. x?=w642:bool)
                                n167 = property on="odd/even indicator" class="Bool (strict)"("Value"=w642) -> ()  [unwired: 2 in, 2 out]
                                }
                                }
                              }
                            }
                            n168 = case shown="True" "acquire 488" {
                              tunnel: w414 -> [w487 w493]
                              tunnel: w412 -> [w485 w497]
                              tunnel: w413 -> [w486 w498]
                              tunnel: [w487 w495] -> _
                              tunnel: [w486 w496] -> _
                              tunnel: [w485 w494] -> _
                              tunnel: w409 -> [_ _]
                              tunnel: w403 -> [_ w490]
                              tunnel: w406 -> [_ w489]
                              tunnel: w400 -> [_ w488]
                              frame False {
                              }
                              frame True {
                                n169 = property on="488 voltages" class="Arr (strict)"() -> ("Value"=w491:dbl[][])  [unwired: 2 in, 2 out]
                                n170 = stacked-sequence {
                                seq-local: [_ w507 _ _] -> [_ _ w528 _]
                                seq-local: [_ w506 _ _] -> [_ _ w527 _]
                                seq-local: [_ w505 _ _] -> [_ _ w523 _]
                                seq-local: [_ w504 _ _] -> [_ _ w521 _]
                                seq-local: [_ w503 _ _] -> [_ _ w520 _]
                                tunnel: w498 -> [_ w507 _ _]
                                tunnel: w497 -> [_ w506 _ _]
                                tunnel: w493 -> [_ w505 _ _]
                                tunnel: w491 -> [_ w504 _ _]
                                tunnel: "488 Exp" -> [_ w503 _ _]
                                tunnel: [_ _ w526 _] -> w496
                                tunnel: [_ _ w525 _] -> w495
                                tunnel: [_ _ w524 _] -> w494
                                tunnel: w491 -> [_ w502 _ _]
                                tunnel: w490 -> [_ w501 _ _]
                                tunnel: w489 -> [w499 _ _ w562]
                                tunnel: w488 -> [_ _ w519 _]
                                frame #0 {
                                n171 = call-poly <vilib>:"DAQmx Write.vi"("task/channels in"=w499, "data"=TRUE) -> ()  [unwired: 11 in, 3 out]
                                }
                                frame #1 {
                                n172 = flat-sequence {
                                tunnel: w502 -> [w514]
                                tunnel: w501 -> [w512]
                                tunnel: [w513] -> _
                                frame #0 {
                                n173 = property on="odd/even indicator" class="Bool (strict)"() -> ("Value"=w508:bool)  [unwired: 2 in, 2 out]
                                n174 = case shown="False" w508 {
                                tunnel: [2 0] -> w510
                                tunnel: [2 0] -> w509
                                frame False {
                                }
                                frame True {
                                }
                                }
                                n175 = Index Array(array=w514, index (row)=w510, index (col)=w509) -> (element=w511:dbl)
                                n176 = call-poly <vilib>:"DAQmx Write.vi"("task/channels in"=w512, "data"=w511) -> ("task out"=w513:refnum<k21>)  [unwired: 11 in, 2 out]
                                }
                                }
                                }
                                frame #2 {
                                n177 = for {
                                N: 9 -> [_]
                                tunnel: w521 -> [w540]
                                tunnel: w523 -> [w538]
                                tunnel: w528 -> [w539]
                                tunnel: w527 -> [w537]
                                tunnel: [w539] -> w526
                                tunnel: [w538] -> w525
                                tunnel: [w537] -> w524
                                tunnel: w520 -> [w536]
                                tunnel: w519 -> [w529]
                                i -> [w535]
                                n178 = property on="odd/even indicator" class="Bool (strict)"() -> ("Value"=w530:bool)  [unwired: 2 in, 2 out]
                                n179 = case shown="True" w530 {
                                tunnel: [i32[] [2, 2, 1, 1, 1, 0, 0, 0, 0, 2, 2, 2, 2, 2, 0] i32[] [0, 0, 1, 1, 1, 2, 2, 2, 2, 2, 2, 2, 2, 2, 0]] -> w531
                                tunnel: [i32[] [1, 0, 2, 1, 0, 2, 1, 0, 0, 0, 1, 2, 3, 4, 0] i32[] [1, 2, 0, 1, 2, 0, 1, 2, 2, 0, 1, 2, 3, 4, 0]] -> w532
                                frame False {
                                }
                                frame True {
                                }
                                }
                                n180 = Index Array(array=w532, index=w535) -> (element=w534:i32)
                                n181 = Index Array(array=w531, index=w535) -> (element=w533:i32)
                                n182 = flat-sequence {
                                tunnel: w540 -> [w549]
                                tunnel: w536 -> [w553]
                                tunnel: w539 -> [w552]
                                tunnel: w538 -> [w551]
                                tunnel: w537 -> [w550]
                                tunnel: w534 -> [w547]
                                tunnel: w533 -> [w546]
                                tunnel: w529 -> [w545]
                                frame #0 {
                                n183 = Index Array(array=w549, index (row)=w547, index (col)=w546) -> (element=w548:dbl)
                                n184 = call "take image.vi"("Voltage"=w548, "Exposure time"=w553, "expose any"=w545, "Busy out"=w550, "Exp In"=w551, "Galvo"=w552) -> ()  [unwired: 6 in]
                                }
                                frame #1 {
                                n185 = property on="Delay time" class="DigNum (strict)"() -> ("Value"=w554:u32)  [unwired: 2 in, 2 out]
                                n186 = Wait (ms)(milliseconds to wait=w554) -> ()  [unwired: 1 out]
                                }
                                }
                                }
                                }
                                frame #3 {
                                n187 = property on="acquire 561" class="Bool (strict)"() -> ("Value"=w558:bool)  [unwired: 2 in, 2 out]
                                n188 = property on="acquire 405" class="Bool (strict)"() -> ("Value"=w557:bool)  [unwired: 2 in, 2 out]
                                n189 = property on="acquire 640" class="Bool (strict)"() -> ("Value"=w559:bool)  [unwired: 2 in, 2 out]
                                n190 = property on="odd/even indicator" class="Bool (strict)"() -> ("Value"=w560:bool)  [unwired: 2 in, 2 out]
                                n191 = Not(x=w560) -> (.not. x?=w561:bool)
                                n192 = Or(x=w558, y=w557) -> (x .or. y?=w556:bool)
                                n193 = property on="odd/even indicator" class="Bool (strict)"("Value"=w561) -> ()  [unwired: 2 in, 2 out]
                                n194 = Or(x=w556, y=w559) -> (x .or. y?=w555:bool)
                                n195 = case shown="True" w555 {
                                tunnel: w562 -> [_ w563]
                                frame False {
                                }
                                frame True {
                                n196 = call-poly <vilib>:"DAQmx Write.vi"("task/channels in"=w563, "data"=FALSE) -> ()  [unwired: 11 in, 3 out]
                                }
                                }
                                }
                                }
                              }
                            }
                            n197 = case shown="True" "acquire 405" {
                              tunnel: w405 -> [_ w428]
                              tunnel: w403 -> [_ w426]
                              tunnel: w402 -> [_ w424]
                              tunnel: w401 -> [_ w423]
                              tunnel: w400 -> [_ w422]
                              frame False {
                              }
                              frame True {
                                n198 = property on="405 voltages" class="Arr (strict)"() -> ("Value"=w427:dbl[][])  [unwired: 2 in, 2 out]
                                n199 = stacked-sequence {
                                tunnel: w427 -> [_ w432 w447 _]
                                tunnel: w426 -> [_ w431 w446 _]
                                tunnel: [_ _ _ w482] -> _
                                tunnel: w428 -> [w429 _ _ w482]
                                tunnel: "405 Exp" -> [_ _ w445 _]
                                tunnel: w424 -> [_ _ w444 _]
                                tunnel: w423 -> [_ _ w443 _]
                                tunnel: w422 -> [_ _ w442 _]
                                frame #0 {
                                n200 = call-poly <vilib>:"DAQmx Write.vi"("task/channels in"=w429, "data"=TRUE) -> ()  [unwired: 11 in, 3 out]
                                }
                                frame #1 {
                                n201 = flat-sequence {
                                tunnel: w432 -> [w436]
                                tunnel: [w435] -> w433
                                tunnel: w431 -> [w434]
                                tunnel: [w441] -> _
                                tunnel: w433 -> [w441]
                                frame #0 {
                                n202 = Index Array(array=w436, index (row)=0, index (col)=0) -> (element=w437:dbl)
                                n203 = call-poly <vilib>:"DAQmx Write.vi"("task/channels in"=w434, "data"=w437) -> ("task out"=w435:refnum<k21>)  [unwired: 11 in, 2 out]
                                }
                                frame #1 {
                                n204 = Wait (ms)(milliseconds to wait=50) -> ()  [unwired: 1 out]
                                }
                                }
                                }
                                frame #2 {
                                n205 = for {
                                N: 9 -> [_]
                                tunnel: w447 -> [w458]
                                tunnel: w446 -> [w457]
                                tunnel: w445 -> [w456]
                                tunnel: w444 -> [w455]
                                tunnel: w443 -> [w454]
                                tunnel: w442 -> [w449]
                                i -> [w453]
                                n206 = property on="odd/even indicator" class="Bool (strict)"() -> ("Value"=w450:bool)  [unwired: 2 in, 2 out]
                                n207 = case shown="True" w450 {
                                tunnel: [i32[] [2, 2, 1, 1, 1, 0, 0, 0, 0, 2, 2, 2, 2, 2, 0] i32[] [0, 0, 1, 1, 1, 2, 2, 2, 2, 2, 2, 2, 2, 2, 0]] -> w452
                                tunnel: [i32[] [1, 0, 2, 1, 0, 2, 1, 0, 0, 0, 1, 2, 3, 4, 0] i32[] [1, 2, 0, 1, 2, 0, 1, 2, 2, 0, 1, 2, 3, 4, 0]] -> w451
                                frame False {
                                }
                                frame True {
                                }
                                }
                                n208 = flat-sequence {
                                tunnel: w460 -> [w472]
                                tunnel: w459 -> [w471]
                                tunnel: w458 -> [w470]
                                tunnel: w457 -> [w469]
                                tunnel: w456 -> [w468]
                                tunnel: w455 -> [w467]
                                tunnel: w454 -> [w466]
                                tunnel: w449 -> [w465]
                                frame #0 {
                                n209 = Index Array(array=w470, index (row)=w472, index (col)=w471) -> (element=w473:dbl)
                                n210 = call "take image.vi"("Voltage"=w473, "Exposure time"=w468, "expose any"=w465, "Busy out"=w466, "Exp In"=w467, "Galvo"=w469) -> ()  [unwired: 6 in]
                                }
                                frame #1 {
                                n211 = property on="Delay time" class="DigNum (strict)"() -> ("Value"=w474:u32)  [unwired: 2 in, 2 out]
                                n212 = Wait (ms)(milliseconds to wait=w474) -> ()  [unwired: 1 out]
                                }
                                }
                                n213 = Index Array(array=w451, index=w453) -> (element=w460:i32)
                                n214 = Index Array(array=w452, index=w453) -> (element=w459:i32)
                                }
                                }
                                frame #3 {
                                n215 = property on="acquire 561" class="Bool (strict)"() -> ("Value"=w477:bool)  [unwired: 2 in, 2 out]
                                n216 = property on="acquire 488" class="Bool (strict)"() -> ("Value"=w478:bool)  [unwired: 2 in, 2 out]
                                n217 = property on="acquire 640" class="Bool (strict)"() -> ("Value"=w476:bool)  [unwired: 2 in, 2 out]
                                n218 = Or(x=w477, y=w478) -> (x .or. y?=w479:bool)
                                n219 = property on="odd/even indicator" class="Bool (strict)"() -> ("Value"=w481:bool)  [unwired: 2 in, 2 out]
                                n220 = Or(x=w479, y=w476) -> (x .or. y?=w475:bool)
                                n221 = Not(x=w481) -> (.not. x?=w480:bool)
                                n222 = property on="odd/even indicator" class="Bool (strict)"("Value"=w480) -> ()  [unwired: 2 in, 2 out]
                                n223 = case shown="True" w475 {
                                tunnel: w482 -> [_ w483]
                                frame False {
                                }
                                frame True {
                                n224 = call-poly <vilib>:"DAQmx Write.vi"("task/channels in"=w483, "data"=FALSE) -> ()  [unwired: 11 in, 3 out]
                                }
                                }
                                }
                                }
                              }
                            }
                          }
                          frame "fast sequence" {
                            # "561"
                            # "488"
                            # "fast sequence"
                            n225 = property on="647 Exp" class="DigNum (strict)"() -> ("Value"=w733:dbl)  [unwired: 2 in, 2 out]
                            n226 = property on="647 voltages" class="Arr (strict)"() -> ("Value"=w736:dbl[][])  [unwired: 2 in, 2 out]
                            n227 = stacked-sequence {
                              seq-local: [_ w818 _ _] -> [_ _ w836 _]
                              seq-local: [_ w817 _ _] -> [_ _ w835 _]
                              seq-local: [_ w816 _ _] -> [_ _ w834 _]
                              seq-local: [_ w815 _ _] -> [_ _ w830 _]
                              seq-local: [_ w814 _ _] -> [_ _ w829 _]
                              tunnel: w744 -> [_ w818 _ _]
                              tunnel: w739 -> [_ w817 _ _]
                              tunnel: w743 -> [_ w816 _ _]
                              tunnel: w736 -> [_ w815 _ _]
                              tunnel: w733 -> [_ w814 _ _]
                              tunnel: [_ _ w833 _] -> w741
                              tunnel: [_ _ w832 _] -> w740
                              tunnel: [_ _ w831 _] -> w742
                              tunnel: w736 -> [_ w812 _ _]
                              tunnel: w739 -> [_ w811 _ _]
                              tunnel: w738 -> [w809 _ _ w867]
                              tunnel: w732 -> [w807 _ _ w865]
                              tunnel: w730 -> [_ _ w827 _]
                              frame #0 {
                                n228 = VISA Write(VISA resource name=w809, write buffer="la on\r" ("format string")) -> ()  [unwired: 1 in, 3 out]
                                n229 = call-poly <vilib>:"DAQmx Write.vi"("task/channels in"=w807, "data"=TRUE) -> ()  [unwired: 11 in, 3 out]
                              }
                              frame #1 {
                                n230 = flat-sequence {
                                tunnel: [w819] -> _
                                tunnel: w812 -> [w821]
                                tunnel: [w820] -> w813
                                tunnel: w811 -> [w819]
                                tunnel: [w826] -> _
                                tunnel: w813 -> [w826]
                                frame #0 {
                                n231 = Index Array(array=w821, index (row)=0, index (col)=0) -> (element=w822:dbl)
                                n232 = call-poly <vilib>:"DAQmx Write.vi"("task/channels in"=w819, "data"=w822) -> ("task out"=w820:refnum<k21>)  [unwired: 11 in, 2 out]
                                }
                                frame #1 {
                                n233 = Wait (ms)(milliseconds to wait=50) -> ()  [unwired: 1 out]
                                }
                                }
                              }
                              frame #2 {
                                n234 = for {
                                N: 9 -> [_]
                                tunnel: w830 -> [w848]
                                tunnel: w836 -> [w845]
                                tunnel: w835 -> [w846]
                                tunnel: w834 -> [w844]
                                tunnel: w829 -> [w847]
                                tunnel: [w846] -> w833
                                tunnel: [w845] -> w832
                                tunnel: [w844] -> w831
                                tunnel: w827 -> [w837]
                                i -> [w842]
                                n235 = property on="odd/even indicator" class="Bool (strict)"() -> ("Value"=w840:bool)  [unwired: 2 in, 2 out]
                                n236 = case shown="False" w840 {
                                tunnel: [i32[] [2, 2, 1, 1, 1, 0, 0, 0, 0, 2, 2, 2, 2, 2, 0] i32[] [0, 0, 1, 1, 1, 2, 2, 2, 2, 2, 2, 2, 2, 2, 0]] -> w838
                                tunnel: [i32[] [1, 0, 2, 1, 0, 2, 1, 0, 0, 0, 1, 2, 3, 4, 0] i32[] [1, 2, 0, 1, 2, 0, 1, 2, 2, 0, 1, 2, 3, 4, 0]] -> w839
                                frame False {
                                }
                                frame True {
                                }
                                }
                                n237 = Index Array(array=w839, index=w842) -> (element=w843:i32)
                                n238 = flat-sequence {
                                tunnel: w848 -> [w857]
                                tunnel: w847 -> [w861]
                                tunnel: w846 -> [w860]
                                tunnel: w845 -> [w859]
                                tunnel: w844 -> [w858]
                                tunnel: w841 -> [w855]
                                tunnel: w843 -> [w854]
                                tunnel: w837 -> [w853]
                                frame #0 {
                                n239 = Index Array(array=w857, index (row)=w854, index (col)=w855) -> (element=w856:dbl)
                                n240 = call "take image.vi"("Voltage"=w856, "Exposure time"=w861, "expose any"=w853, "Busy out"=w858, "Exp In"=w859, "Galvo"=w860) -> ()  [unwired: 6 in]
                                }
                                frame #1 {
                                n241 = property on="Delay time" class="DigNum (strict)"() -> ("Value"=w862:u32)  [unwired: 2 in, 2 out]
                                n242 = Wait (ms)(milliseconds to wait=w862) -> ()  [unwired: 1 out]
                                }
                                }
                                n243 = Index Array(array=w838, index=w842) -> (element=w841:i32)
                                }
                              }
                              frame #3 {
                                n244 = property on="odd/even indicator" class="Bool (strict)"() -> ("Value"=w863:bool)  [unwired: 2 in, 2 out]
                                n245 = Not(x=w863) -> (.not. x?=w864:bool)
                                n246 = property on="odd/even indicator" class="Bool (strict)"("Value"=w864) -> ()  [unwired: 2 in, 2 out]
                                n247 = VISA Write(VISA resource name=w867, write buffer="la off\r" ("format string")) -> ()  [unwired: 1 in, 3 out]
                                n248 = call-poly <vilib>:"DAQmx Write.vi"("task/channels in"=w865, "data"=FALSE) -> ()  [unwired: 11 in, 3 out]
                              }
                            }
                            n249 = property on="561 voltages" class="Arr (strict)"() -> ("Value"=w735:dbl[][])  [unwired: 2 in, 2 out]
                            n250 = property on="561 Exp" class="DigNum (strict)"() -> ("Value"=w734:dbl)  [unwired: 2 in, 2 out]
                            n251 = stacked-sequence {
                              seq-local: [_ w756 _ _] -> [_ _ w774 _]
                              seq-local: [_ w755 _ _] -> [_ _ w773 _]
                              seq-local: [_ w754 _ _] -> [_ _ w769 _]
                              seq-local: [_ w753 _ _] -> [_ _ w767 _]
                              seq-local: [_ w752 _ _] -> [_ _ w766 _]
                              tunnel: w741 -> [_ w756 _ _]
                              tunnel: w742 -> [_ w755 _ _]
                              tunnel: w740 -> [_ w754 _ _]
                              tunnel: w735 -> [_ w753 _ _]
                              tunnel: w734 -> [_ w752 _ _]
                              tunnel: [_ _ w772 _] -> _
                              tunnel: [_ _ w771 _] -> _
                              tunnel: [_ _ w770 _] -> _
                              tunnel: w735 -> [_ w750 _ _]
                              tunnel: w739 -> [_ w749 _ _]
                              tunnel: w737 -> [w748 _ _ w805]
                              tunnel: w731 -> [w745 _ _ w803]
                              tunnel: w730 -> [_ _ w765 _]
                              frame #0 {
                                n252 = call-poly <vilib>:"DAQmx Write.vi"("task/channels in"=w748, "data"=TRUE) -> ()  [unwired: 11 in, 3 out]
                                n253 = call-poly <vilib>:"DAQmx Write.vi"("task/channels in"=w745, "data"=TRUE) -> ()  [unwired: 11 in, 3 out]
                              }
                              frame #1 {
                                n254 = flat-sequence {
                                tunnel: w750 -> [w759]
                                tunnel: [w758] -> w751
                                tunnel: w749 -> [w757]
                                tunnel: [w764] -> _
                                tunnel: w751 -> [w764]
                                frame #0 {
                                n255 = Index Array(array=w759, index (row)=0, index (col)=0) -> (element=w760:dbl)
                                n256 = call-poly <vilib>:"DAQmx Write.vi"("task/channels in"=w757, "data"=w760) -> ("task out"=w758:refnum<k21>)  [unwired: 11 in, 2 out]
                                }
                                frame #1 {
                                n257 = Wait (ms)(milliseconds to wait=50) -> ()  [unwired: 1 out]
                                }
                                }
                              }
                              frame #2 {
                                n258 = for {
                                N: 9 -> [_]
                                tunnel: w767 -> [w786]
                                tunnel: w769 -> [w783]
                                tunnel: w774 -> [w784]
                                tunnel: w773 -> [w782]
                                tunnel: w766 -> [w785]
                                tunnel: [w784] -> w772
                                tunnel: [w783] -> w771
                                tunnel: [w782] -> w770
                                tunnel: w765 -> [w775]
                                i -> [w781]
                                n259 = property on="odd/even indicator" class="Bool (strict)"() -> ("Value"=w776:bool)  [unwired: 2 in, 2 out]
                                n260 = case shown="True" w776 {
                                tunnel: [i32[] [2, 2, 1, 1, 1, 0, 0, 0, 0, 2, 2, 2, 2, 2, 0] i32[] [0, 0, 1, 1, 1, 2, 2, 2, 2, 2, 2, 2, 2, 2, 0]] -> w777
                                tunnel: [i32[] [1, 0, 2, 1, 0, 2, 1, 0, 0, 0, 1, 2, 3, 4, 0] i32[] [1, 2, 0, 1, 2, 0, 1, 2, 2, 0, 1, 2, 3, 4, 0]] -> w778
                                frame False {
                                }
                                frame True {
                                }
                                }
                                n261 = Index Array(array=w778, index=w781) -> (element=w780:i32)
                                n262 = Index Array(array=w777, index=w781) -> (element=w779:i32)
                                n263 = flat-sequence {
                                tunnel: w786 -> [w795]
                                tunnel: w785 -> [w799]
                                tunnel: w784 -> [w798]
                                tunnel: w783 -> [w797]
                                tunnel: w782 -> [w796]
                                tunnel: w780 -> [w793]
                                tunnel: w779 -> [w792]
                                tunnel: w775 -> [w791]
                                frame #0 {
                                n264 = Index Array(array=w795, index (row)=w793, index (col)=w792) -> (element=w794:dbl)
                                n265 = call "take image.vi"("Voltage"=w794, "Exposure time"=w799, "expose any"=w791, "Busy out"=w796, "Exp In"=w797, "Galvo"=w798) -> ()  [unwired: 6 in]
                                }
                                frame #1 {
                                n266 = property on="Delay time" class="DigNum (strict)"() -> ("Value"=w800:u32)  [unwired: 2 in, 2 out]
                                n267 = Wait (ms)(milliseconds to wait=w800) -> ()  [unwired: 1 out]
                                }
                                }
                                }
                              }
                              frame #3 {
                                n268 = call-poly <vilib>:"DAQmx Write.vi"("task/channels in"=w805, "data"=FALSE) -> ()  [unwired: 11 in, 3 out]
                                n269 = property on="odd/even indicator" class="Bool (strict)"() -> ("Value"=w802:bool)  [unwired: 2 in, 2 out]
                                n270 = call-poly <vilib>:"DAQmx Write.vi"("task/channels in"=w803, "data"=FALSE) -> ()  [unwired: 11 in, 3 out]
                                n271 = Not(x=w802) -> (.not. x?=w801:bool)
                                n272 = property on="odd/even indicator" class="Bool (strict)"("Value"=w801) -> ()  [unwired: 2 in, 2 out]
                              }
                            }
                          }
                          frame "optosplit" {
                            n273 = case shown="False" w870 {
                              tunnel: w873 -> [w879 w916]
                              tunnel: w872 -> [w878 w915]
                              tunnel: w871 -> [w877 w914]
                              tunnel: w869 -> [_ w908]
                              frame True {
                                w874 = 15
                                # "With optosplit"
                                n274 = flat-sequence {
                                tunnel: w877 -> [w883]
                                tunnel: w876 -> [w882]
                                tunnel: [w881] -> w880
                                tunnel: [w890] -> w875
                                tunnel: w880 -> [w890]
                                frame #0 {
                                n275 = Index Array(array=w882, index (row)=0, index (col)=0) -> (element=w884:dbl)
                                n276 = call-poly <vilib>:"DAQmx Write.vi"("task/channels in"=w883, "data"=w884) -> ("task out"=w881:refnum<k21>)  [unwired: 11 in, 2 out]
                                }
                                frame #1 {
                                n277 = property on="Delay time" class="DigNum (strict)"() -> ("Value"=w889:u32)  [unwired: 2 in, 2 out]
                                n278 = Add(x=w889, y=20) -> (x+y=w888:u32)
                                n279 = Wait (ms)(milliseconds to wait=w888) -> ()  [unwired: 1 out]
                                }
                                }
                                n280 = property on="561 voltages" class="Arr (strict)"() -> ("Value"=w876:dbl[][])  [unwired: 2 in, 2 out]
                                n281 = for {
                                N: w874 -> [_]
                                tunnel: w876 -> [w898]
                                tunnel: w879 -> [w901]
                                tunnel: w878 -> [w900]
                                tunnel: w875 -> [w899]
                                tunnel: w874 -> [_]
                                i -> [w894]
                                n282 = property on="Exposure time" class="DigNum (strict)"() -> ("Value"=w897:dbl)  [unwired: 2 in, 2 out]
                                n283 = Index Array(array=i32[] [1, 2, 3, 4, 0, 1, 2, 3, 4, 0, 1, 2, 3, 4, 0], index=w894) -> (element=w892:i32)
                                n284 = Index Array(array=i32[] [0, 0, 0, 0, 1, 1, 1, 1, 1, 2, 2, 2, 2, 2, 0], index=w894) -> (element=w893:i32)
                                n285 = Index Array(array=w898, index (row)=w892, index (col)=w893) -> (element=w891:dbl)
                                n286 = property on="Current voltage" class="DigNum (strict)"("Value"=w891) -> ()  [unwired: 2 in, 2 out]
                                n287 = flat-sequence {
                                tunnel: w901 -> [w906]
                                tunnel: w900 -> [w905]
                                tunnel: w891 -> [w904]
                                tunnel: w899 -> [w903]
                                tunnel: w897 -> [w902]
                                frame #0 {
                                n288 = call "take image.vi"("Voltage"=w904, "Exposure time"=w902, "Busy out"=w905, "Exp In"=w906, "Galvo"=w903) -> ()  [unwired: 7 in]
                                }
                                frame #1 {
                                n289 = property on="Delay time" class="DigNum (strict)"() -> ("Value"=w907:u32)  [unwired: 2 in, 2 out]
                                n290 = Wait (ms)(milliseconds to wait=w907) -> ()  [unwired: 1 out]
                                }
                                }
                                }
                              }
                              frame False {
                                w911 = 9
                                # "With optosplit"
                                n291 = flat-sequence {
                                tunnel: w914 -> [w923]
                                tunnel: w913 -> [w922]
                                tunnel: [w921] -> w917
                                tunnel: [w932] -> w912
                                tunnel: w917 -> [w932]
                                frame #0 {
                                n292 = property on="odd/even indicator" class="Bool (strict)"() -> ("Value"=w920:bool)  [unwired: 2 in, 2 out]
                                n293 = case shown="False" w920 {
                                tunnel: [2 0] -> w919
                                tunnel: [2 0] -> w918
                                frame False {
                                }
                                frame True {
                                }
                                }
                                n294 = Index Array(array=w922, index (row)=w919, index (col)=w918) -> (element=w924:dbl)
                                n295 = call-poly <vilib>:"DAQmx Write.vi"("task/channels in"=w923, "data"=w924) -> ("task out"=w921:refnum<k21>)  [unwired: 11 in, 2 out]
                                }
                                frame #1 {
                                n296 = property on="Delay time" class="DigNum (strict)"() -> ("Value"=w931:u32)  [unwired: 2 in, 2 out]
                                n297 = Add(x=w931, y=20) -> (x+y=w930:u32)
                                n298 = Wait (ms)(milliseconds to wait=w930) -> ()  [unwired: 1 out]
                                }
                                }
                                n299 = property on="561 voltages" class="Arr (strict)"() -> ("Value"=w913:dbl[][])  [unwired: 2 in, 2 out]
                                n300 = for {
                                N: w911 -> [_]
                                tunnel: w913 -> [w942]
                                tunnel: w916 -> [w945]
                                tunnel: w915 -> [w944]
                                tunnel: w912 -> [w943]
                                tunnel: w911 -> [_]
                                tunnel: [w934] -> w909
                                tunnel: w908 -> [w933]
                                i -> [w940]
                                n301 = property on="odd/even indicator" class="Bool (strict)"() -> ("Value"=w934:bool)  [unwired: 2 in, 2 out]
                                n302 = property on="Exposure time" class="DigNum (strict)"() -> ("Value"=w941:dbl)  [unwired: 2 in, 2 out]
                                n303 = case shown="False" w934 {
                                tunnel: [i32[] [2, 2, 1, 1, 1, 0, 0, 0, 0, 2, 2, 2, 2, 2, 0] i32[] [0, 0, 1, 1, 1, 2, 2, 2, 2, 2, 2, 2, 2, 2, 0]] -> w935
                                tunnel: [i32[] [1, 0, 2, 1, 0, 2, 1, 0, 0, 0, 1, 2, 3, 4, 0] i32[] [1, 2, 0, 1, 2, 0, 1, 2, 2, 0, 1, 2, 3, 4, 0]] -> w936
                                frame False {
                                }
                                frame True {
                                }
                                }
                                n304 = Index Array(array=w936, index=w940) -> (element=w938:i32)
                                n305 = Index Array(array=w935, index=w940) -> (element=w939:i32)
                                n306 = Index Array(array=w942, index (row)=w938, index (col)=w939) -> (element=w937:dbl)
                                n307 = property on="Current voltage" class="DigNum (strict)"("Value"=w937) -> ()  [unwired: 2 in, 2 out]
                                n308 = flat-sequence {
                                tunnel: w945 -> [w955]
                                tunnel: w944 -> [w954]
                                tunnel: w937 -> [w953]
                                tunnel: w943 -> [w952]
                                tunnel: w941 -> [w951]
                                tunnel: w933 -> [w950]
                                frame #0 {
                                n309 = call "take image.vi"("Voltage"=w953, "Exposure time"=w951, "expose any"=w950, "Busy out"=w954, "Exp In"=w955, "Galvo"=w952) -> ()  [unwired: 6 in]
                                }
                                frame #1 {
                                n310 = property on="Delay time" class="DigNum (strict)"() -> ("Value"=w956:u32)  [unwired: 2 in, 2 out]
                                n311 = Wait (ms)(milliseconds to wait=w956) -> ()  [unwired: 1 out]
                                }
                                }
                                }
                                n312 = Not(x=w909) -> (.not. x?=w910:bool)
                                n313 = property on="odd/even indicator" class="Bool (strict)"("Value"=w910) -> ()  [unwired: 2 in, 2 out]
                              }
                            }
                          }
                          frame "rolling SIM" {
                            w960 = 0 ("index")
                            # "Rolling SIM"
                            n314 = Build Array("short delay", "short delay", "long delay") -> (w961:dbl[])
                            n315 = Insert Into Array(array=w961, index=w960, new element=w961) -> (w962:dbl[])
                            n316 = Insert Into Array(array=w962, index=w960, new element=w962) -> (w957:dbl[])
                            n317 = property on="561 voltages" class="Arr (strict)"() -> ("Value"=w968:dbl[][])  [unwired: 2 in, 2 out]
                            n318 = for {
                              N: 12 -> [_]
                              tunnel: w968 -> [w973]
                              tunnel: w970 -> [w984]
                              tunnel: w969 -> [w983]
                              tunnel: [w976] -> w965
                              tunnel: w964 -> [w975]
                              tunnel: w963 -> [w974]
                              tunnel: w957 -> [w971] mode=indexing
                              i -> [w972]
                              n319 = property on="Exposure time" class="DigNum (strict)"() -> ("Value"=w982:dbl)  [unwired: 2 in, 2 out]
                              n320 = Index Array(array=i32[] [1, 2, 0, 1, 2, 0, 1, 2, 2, 1, 0, 0, 3, 4, 0], index=w972) -> (element=w980:i32)
                              n321 = Index Array(array=i32[] [0, 0, 1, 1, 1, 2, 2, 2, 1, 1, 1, 0, 2, 2, 0], index=w972) -> (element=w981:i32)
                              n322 = Index Array(array=w973, index (row)=w980, index (col)=w981) -> (element=w979:dbl)
                              n323 = property on="Current voltage" class="DigNum (strict)"("Value"=w979) -> ()  [unwired: 2 in, 2 out]
                              n324 = flat-sequence {
                                tunnel: w984 -> [w990]
                                tunnel: w983 -> [w986]
                                tunnel: w979 -> [w989]
                                tunnel: w982 -> [w988]
                                tunnel: w975 -> [w987]
                                tunnel: w974 -> [w985]
                                tunnel: w971 -> [w991]
                                frame #0 {
                                n325 = call "take image.vi"("Voltage"=w989, "Exposure time"=w988, "expose any"=w987, "Busy out"=w986, "Exp In"=w990, "Galvo"=w985) -> ()  [unwired: 6 in]
                                }
                                frame #1 {
                                n326 = Wait (ms)(milliseconds to wait=w991) -> ()  [unwired: 1 out]
                                }
                              }
                              n327 = property on="odd/even indicator" class="Bool (strict)"() -> ("Value"=w976:bool)  [unwired: 2 in, 2 out]
                            }
                            n328 = Not(x=w965) -> (.not. x?=w966:bool)
                            n329 = property on="odd/even indicator" class="Bool (strict)"("Value"=w966) -> ()  [unwired: 2 in, 2 out]
                          }
                        }
                      }
                      frame #1 {
                        n330 = Greater?(x=w995, y=1) -> (0:w994:bool)
                        n331 = Greater?(x="Steps /um", y=0) -> (0:w993:bool)
                        n332 = And(x=w994, y=w993) -> (x .and. y?=w992:bool)
                        n333 = case shown="True" w992 {
                          tunnel: w1000 -> [w1001 w1004]
                          tunnel: [w1001 w1003] -> w999
                          tunnel: "Steps /um" -> [_ w1002]
                          frame False {
                          }
                          frame True {
                            n334 = flat-sequence {
                              tunnel: w1004 -> [w1012]
                              tunnel: [w1011] -> w1005
                              tunnel: w1002 -> [w1008]
                              tunnel: [w1015] -> w1003
                              tunnel: w1005 -> [w1015]
                              frame #0 {
                                n335 = Multiply(x=w1008, y=10.0) -> (x*y=w1006:dbl)
                                n336 = Format Into String "Format Into String"(format string="movrel\\sz=%f\\s\\r\\n", w1006) -> (resulting string=w1009:string)  [unwired: 2 in, 1 out]
                                "resulting string" <- w1009
                                n337 = VISA Write(VISA resource name=w1012, write buffer=w1009) -> (VISA resource name out=w1011:refnum<visa-resource-name>, error out=→"optosplit stage error":errorcluster)  [unwired: 1 in, 1 out]
                              }
                              frame #1 {
                                n338 = Wait (ms)(milliseconds to wait=20) -> ()  [unwired: 1 out]
                              }
                            }
                          }
                        }
                      }
                    }
                  }
                }
                frame #1 {
                  n339 = flat-sequence {
                    tunnel: w1031 -> [w1041]
                    tunnel: w1030 -> [w1040]
                    tunnel: w1029 -> [w1039]
                    tunnel: w1028 -> [w1038]
                    tunnel: [w1037] -> w1025
                    tunnel: [w1036] -> w1022
                    tunnel: [w1035] -> w1019
                    tunnel: [w1034] -> w1018
                    tunnel: w1032 -> [w1065]
                    tunnel: [w1064] -> w1026
                    tunnel: w1025 -> [w1064]
                    tunnel: [w1063] -> w1023
                    tunnel: w1022 -> [w1063]
                    tunnel: [w1062] -> w1020
                    tunnel: w1019 -> [w1062]
                    tunnel: w1018 -> [w1061]
                    tunnel: [w1061] -> w1016
                    tunnel: [w1079] -> w1027
                    tunnel: w1026 -> [w1079]
                    tunnel: [w1078] -> w1024
                    tunnel: w1023 -> [w1078]
                    tunnel: [w1077] -> w1021
                    tunnel: w1020 -> [w1077]
                    tunnel: [w1076] -> w1017
                    tunnel: w1016 -> [w1076]
                    tunnel: w1027 -> [w1086]
                    tunnel: w1024 -> [w1085]
                    tunnel: w1021 -> [w1084]
                    tunnel: w1017 -> [w1083]
                    frame #0 {
                      n340 = case shown="False" FALSE {
                        tunnel: w1041 -> [w1045 w1053]
                        tunnel: w1040 -> [w1044 w1052]
                        tunnel: w1039 -> [w1043 w1051]
                        tunnel: w1038 -> [w1042 w1050]
                        tunnel: [w1042 w1049] -> w1037
                        tunnel: [w1043 w1048] -> w1036
                        tunnel: [w1044 w1047] -> w1035
                        tunnel: [w1045 w1046] -> w1034
                        frame False {
                        }
                        frame True {
                          n341 = call-poly <vilib>:"DAQmx Write.vi"("task/channels in"=w1052, "data"=FALSE) -> ("task out"=w1047:refnum<k21>)  [unwired: 11 in, 2 out]
                          n342 = call-poly <vilib>:"DAQmx Write.vi"("task/channels in"=w1053, "data"=FALSE) -> ("task out"=w1046:refnum<k21>)  [unwired: 11 in, 2 out]
                          n343 = call-poly <vilib>:"DAQmx Write.vi"("task/channels in"=w1051, "data"=FALSE) -> ("task out"=w1048:refnum<k21>)  [unwired: 11 in, 2 out]
                          n344 = VISA Write(VISA resource name=w1050, write buffer="la off\r" ("format string")) -> (VISA resource name out=w1049:refnum<visa-resource-name>)  [unwired: 1 in, 2 out]
                        }
                      }
                    }
                    frame #1 {
                      n345 = property on="z-slices" class="DigNum (strict)"() -> ("Value"=w1059:dbl)  [unwired: 2 in, 2 out]
                      n346 = property on="Optosplit" class="RadioBtnsControl (strict)" props=["Value"]() -> ()  [unwired: 2 in, 3 out]
                      n347 = Greater?(x=w1059, y=1) -> (0:w1058:bool)
                      n348 = case shown="False" w1058 {
                        tunnel: w1065 -> [_ w1072]
                        frame False {
                        }
                        frame True {
                          n349 = property on="z-slices" class="DigNum (strict)"() -> ("Value"=w1070:dbl)  [unwired: 2 in, 2 out]
                          n350 = property on="Steps /um" class="DigNum (strict)"() -> ("Value"=w1071:dbl)  [unwired: 2 in, 2 out]
                          n351 = Negate(x=w1071) -> (-x=w1069:dbl)
                          n352 = Multiply(x=w1069, y=w1070) -> (x*y=w1068:dbl)
                          n353 = Multiply(x=w1068, y=10.0) -> (x*y=w1066:dbl)
                          n354 = Format Into String "Format Into String"(format string="movrel\\sz=%f\\s\\r\\n", w1066) -> (resulting string=w1074:string)  [unwired: 2 in, 1 out]
                          "resulting string 2" <- w1074
                          n355 = VISA Write(VISA resource name=w1072, write buffer=w1074) -> (error out=→"stage error":errorcluster)  [unwired: 1 in, 2 out]
                        }
                      }
                    }
                    frame #2 {
                      n356 = Multiply(x="interval /s", y=1000.0) -> (x*y=w1082:dbl)
                      n357 = Wait (ms)(milliseconds to wait=w1082) -> ()  [unwired: 1 out]
                    }
                    frame #3 {
                      n358 = property on="Optosplit" class="RadioBtnsControl (strict)"() -> ("Value"=w1087:T3)  [unwired: 2 in, 2 out]
                      n359 = disable-structure shown="Disabled" {
                        disable-tunnel: w1087 -> [w1092 _]
                        disable-tunnel: w1086 -> [w1091 _]
                        disable-tunnel: w1085 -> [w1090 _]
                        disable-tunnel: w1084 -> [w1089 _]
                        disable-tunnel: w1083 -> [w1088 _]
                        frame Disabled {
                          n360 = case shown="\"rolling SIM\"" w1092 {
                            tunnel: w1091 -> [_ w1096 w1104 w1112]
                            tunnel: w1090 -> [_ w1095 w1103 w1111]
                            tunnel: w1089 -> [_ w1094 w1102 w1110]
                            tunnel: w1088 -> [_ w1093 w1101 w1109]
                            frame "sequential", Default {
                            }
                            frame "optosplit" {
                              n361 = call-poly <vilib>:"DAQmx Write.vi"("task/channels in"=w1094, "data"=TRUE) -> ()  [unwired: 11 in, 3 out]
                              n362 = call-poly <vilib>:"DAQmx Write.vi"("task/channels in"=w1093, "data"=TRUE) -> ()  [unwired: 11 in, 3 out]
                              n363 = call-poly <vilib>:"DAQmx Write.vi"("task/channels in"=w1095, "data"=TRUE) -> ()  [unwired: 11 in, 3 out]
                              n364 = VISA Write(VISA resource name=w1096, write buffer="la on\r" ("format string")) -> ()  [unwired: 1 in, 3 out]
                            }
                            frame "rolling SIM" {
                              n365 = call-poly <vilib>:"DAQmx Write.vi"("task/channels in"=w1102, "data"=TRUE) -> ()  [unwired: 11 in, 3 out]
                              n366 = call-poly <vilib>:"DAQmx Write.vi"("task/channels in"=w1101, "data"=TRUE) -> ()  [unwired: 11 in, 3 out]
                              n367 = call-poly <vilib>:"DAQmx Write.vi"("task/channels in"=w1103, "data"=TRUE) -> ()  [unwired: 11 in, 3 out]
                              n368 = VISA Write(VISA resource name=w1104, write buffer="la on\r" ("format string")) -> ()  [unwired: 1 in, 3 out]
                            }
                            frame "fast sequence" {
                              n369 = call-poly <vilib>:"DAQmx Write.vi"("task/channels in"=w1110, "data"=TRUE) -> ()  [unwired: 11 in, 3 out]
                              n370 = call-poly <vilib>:"DAQmx Write.vi"("task/channels in"=w1109, "data"=TRUE) -> ()  [unwired: 11 in, 3 out]
                              n371 = call-poly <vilib>:"DAQmx Write.vi"("task/channels in"=w1111, "data"=TRUE) -> ()  [unwired: 11 in, 3 out]
                              n372 = VISA Write(VISA resource name=w1112, write buffer="la on\r" ("format string")) -> ()  [unwired: 1 in, 3 out]
                            }
                          }
                        }
                        frame Enabled {
                        }
                      }
                    }
                  }
                }
              }
              n373 = property on="Go SIM" class="Bool (strict)"() -> ("Value"=w332:bool)  [unwired: 2 in, 2 out]
              n374 = Not(x=w332) -> (.not. x?=w331:bool)
            }
          }
          frame #3 {
            w1118 = FALSE
            n375 = property on="Tab Control" class="TabCtl (strict)"("DisabledEnum"=T5."Enabled" ("Disabled")) -> ()  [unwired: 2 in, 2 out]
            n376 = call-poly <vilib>:"DAQmx Write.vi"("task/channels in"=w1121, "data"=FALSE) -> ()  [unwired: 11 in, 3 out]
            n377 = call-poly <vilib>:"DAQmx Write.vi"("task/channels in"=w1122, "data"=FALSE) -> ()  [unwired: 11 in, 3 out]
            n378 = VISA Write(VISA resource name=w1119, write buffer="la off\r" ("format string")) -> ()  [unwired: 1 in, 3 out]
            n379 = property on="561" class="Bool (strict)"("Value"=w1118) -> ()  [unwired: 2 in, 2 out]
            n380 = property on="488" class="Bool (strict)"("Value"=w1118) -> ()  [unwired: 2 in, 2 out]
            n381 = property on="405" class="Bool (strict)"("Value"=w1118) -> ()  [unwired: 2 in, 2 out]
            n382 = property on="647" class="Bool (strict)"("Value"=w1118) -> ()  [unwired: 2 in, 2 out]
          }
        }
      }
    }
    n383 = property on="stop" class="Bool (strict)"() -> ("Value"=w158:bool)  [unwired: 2 in, 2 out]
  }
  n384 = VISA Write(VISA resource name=w27, write buffer="en 1\r" ("format string")) -> (VISA resource name out=w26:refnum<visa-resource-name>)  [unwired: 1 in, 2 out]
  n385 = property class="MG17Motor"(reference="MG17Motor", "HWSerialNum"=i64 83839541 ("Numeric 2")) -> (reference out=w34:refnum<k7>)  [unwired: 1 in, 1 out]
  n386 = invoke class="MG17Motor" method="StartCtrl"(reference=w34) -> (reference out=w33:refnum<k7>, error out=w32:errorcluster)  [unwired: 2 in, 1 out]
  n387 = while {
    tunnel: w1 -> [w1136]
    tunnel: w3 -> [w1135]
    tunnel: w2 -> [w1137]
    tunnel: ["stop"] -> _
    tunnel: [w1137] -> w68
    tunnel: [w1136] -> w67
    tunnel: [w1135] -> w69
    shift-right: [w1129] -> _
    shift-left: 0 -> [w1128]
    tunnel: w10 -> [w1126]
    tunnel: [w1126] -> w9
    stop <- "stop" stop-if-true
    n388 = Greater?(x=w1128, y=8) -> (0:w1131:bool)
    n389 = Select(t=0, s=w1131, f=w1128) -> (s? t:f=w1130:i32)
    n390 = Add(x=1, y=w1130) -> (x+y=w1129:i32)
    "x+y" <- w1129
    n391 = case shown="True" "Go live" {
      tunnel: w1137 -> [_ w1144]
      tunnel: w1136 -> [_ w1143]
      tunnel: w1135 -> [_ w1142]
      tunnel: w1129 -> [_ w1139]
      frame False {
      }
      frame True {
        n392 = property on="561 voltages" class="Arr (strict)"() -> ("Value"=w1140:dbl[][])  [unwired: 2 in, 2 out]
        n393 = case shown="\"Mirror 1\", Default" "Live mode" {
          tunnel: w1140 -> [w1159 w1202 w1252 w1298 w1329 w1363]
          tunnel: w1143 -> [w1160 w1199 w1238 w1299 w1323 w1362]
          tunnel: w1142 -> [w1147 w1185 w1240 w1286 _ w1361]
          tunnel: w1144 -> [w1146 w1186 w1239 w1285 _ w1356]
          tunnel: w1139 -> [_ _ w1228 _ _ _]
          frame "Mirror 1", Default {
            n394 = Index Array(array=w1159, index (row)=2, index (col)=0) -> (element=w1158:dbl)
            n395 = call-poly <vilib>:"DAQmx Write.vi"("task/channels in"=w1160, "data"=w1158) -> ("error out"=w1145:errorcluster)  [unwired: 11 in, 2 out]
            n396 = flat-sequence {
              tunnel: w1147 -> [w1166]
              tunnel: [w1164] -> w1155
              tunnel: w1145 -> [w1163]
              tunnel: [w1162] -> w1154
              tunnel: w1146 -> [w1161]
              tunnel: [w1161] -> w1153
              tunnel: w1155 -> [w1170]
              tunnel: [w1170] -> w1152
              tunnel: w1154 -> [w1168]
              tunnel: [w1169] -> w1151
              tunnel: w1153 -> [w1169]
              tunnel: [w1168] -> w1150
              tunnel: w1152 -> [w1175]
              tunnel: [w1173] -> w1149
              tunnel: w1151 -> [w1173]
              tunnel: w1150 -> [w1172]
              tunnel: [w1171] -> w1148
              tunnel: w1149 -> [w1178]
              tunnel: w1148 -> [w1177]
              tunnel: [w1176] -> _
              frame #0 {
                n397 = call-poly <vilib>:"DAQmx Write.vi"("task/channels in"=w1166, "data"=TRUE, "error in"=w1163) -> ("task out"=w1164:refnum<k21>, "error out"=w1162:errorcluster)  [unwired: 10 in, 1 out]
              }
              frame #1 {
                n398 = property on="Exposure time" class="DigNum (strict)"() -> ("Value"=w1167:dbl)  [unwired: 2 in, 2 out]
                n399 = Wait (ms)(milliseconds to wait=w1167) -> ()  [unwired: 1 out]
              }
              frame #2 {
                n400 = call-poly <vilib>:"DAQmx Write.vi"("task/channels in"=w1175, "data"=FALSE, "error in"=w1172) -> ("error out"=w1171:errorcluster)  [unwired: 10 in, 2 out]
              }
              frame #3 {
                n401 = while {
                  tunnel: w1178 -> [w1183]
                  tunnel: w1177 -> [w1182]
                  tunnel: [w1181] -> w1176
                  stop <- w1180 stop-if-true
                  n402 = call-poly <vilib>:"DAQmx Read.vi"("task/channels in"=w1183, "error in"=w1182) -> ("data"=w1179:bool, "error out"=w1181:errorcluster)  [unwired: 11 in, 1 out]
                  n403 = Not(x=w1179) -> (.not. x?=w1180:bool)
                }
              }
            }
          }
          frame "Widefield" {
            n404 = Index Array(array=w1202, index (row)=2, index (col)=1) -> ()  [unwired: 1 out]
            n405 = call <vilib>:"Triangle Waveform.vi"("offset"=1.0, "phase"=0.0, "amplitude"=0.06, "frequency"=0.1) -> ("signal out"=w1195:waveform(dbl))  [unwired: 6 in, 1 out]
            n406 = call-poly <vilib>:"DAQmx Write.vi"("task/channels in"=w1199, "data"=w1195) -> ()  [unwired: 11 in, 3 out]
            n407 = flat-sequence {
              tunnel: w1185 -> [w1207]
              tunnel: [w1205] -> w1194
              tunnel: [w1204] -> w1193
              tunnel: [w1203] -> w1192
              tunnel: w1186 -> [w1203]
              tunnel: w1194 -> [w1211]
              tunnel: [w1211] -> w1191
              tunnel: w1193 -> [w1209]
              tunnel: [w1210] -> w1190
              tunnel: w1192 -> [w1210]
              tunnel: [w1209] -> w1189
              tunnel: w1191 -> [w1216]
              tunnel: [w1214] -> w1188
              tunnel: w1190 -> [w1214]
              tunnel: w1189 -> [w1213]
              tunnel: [w1212] -> w1187
              tunnel: w1188 -> [w1219]
              tunnel: w1187 -> [w1218]
              tunnel: [w1217] -> _
              frame #0 {
                n408 = call-poly <vilib>:"DAQmx Write.vi"("task/channels in"=w1207, "data"=TRUE) -> ("task out"=w1205:refnum<k21>, "error out"=w1204:errorcluster)  [unwired: 11 in, 1 out]
              }
              frame #1 {
                n409 = property on="Exposure time" class="DigNum (strict)"() -> ("Value"=w1208:dbl)  [unwired: 2 in, 2 out]
                n410 = Wait (ms)(milliseconds to wait=w1208) -> ()  [unwired: 1 out]
              }
              frame #2 {
                n411 = call-poly <vilib>:"DAQmx Write.vi"("task/channels in"=w1216, "data"=FALSE, "error in"=w1213) -> ("error out"=w1212:errorcluster)  [unwired: 10 in, 2 out]
              }
              frame #3 {
                n412 = while {
                  tunnel: w1219 -> [w1224]
                  tunnel: w1218 -> [w1223]
                  tunnel: [w1222] -> w1217
                  stop <- w1221 stop-if-true
                  n413 = call-poly <vilib>:"DAQmx Read.vi"("task/channels in"=w1224, "error in"=w1223) -> ("data"=w1220:bool, "error out"=w1222:errorcluster)  [unwired: 11 in, 1 out]
                  n414 = Not(x=w1220) -> (.not. x?=w1221:bool)
                }
              }
            }
          }
          frame "SIM" {
            n415 = Quotient & Remainder(x=w1228, y=9) -> (x-y*floor(x/y)=w1250:i32)  [unwired: 1 out]
            n416 = flat-sequence {
              tunnel: w1239 -> [w1256]
              tunnel: w1240 -> [w1257]
              tunnel: [w1257] -> w1237
              tunnel: [w1253] -> w1235
              tunnel: [w1256] -> w1233
              tunnel: w1238 -> [w1255]
              tunnel: w1227 -> [w1254]
              tunnel: w1237 -> [w1261]
              tunnel: [w1261] -> w1236
              tunnel: w1235 -> [w1260]
              tunnel: [w1260] -> w1234
              tunnel: w1233 -> [w1259]
              tunnel: [w1259] -> w1232
              tunnel: [w1265] -> w1248
              tunnel: [w1263] -> w1247
              tunnel: [w1262] -> w1246
              tunnel: w1236 -> [w1267]
              tunnel: w1234 -> [w1264]
              tunnel: w1232 -> [w1262]
              tunnel: w1248 -> [w1271]
              tunnel: [w1271] -> w1245
              tunnel: w1247 -> [w1269]
              tunnel: [w1270] -> w1244
              tunnel: w1246 -> [w1270]
              tunnel: [w1269] -> w1243
              tunnel: w1245 -> [w1276]
              tunnel: [w1274] -> w1242
              tunnel: w1244 -> [w1274]
              tunnel: w1243 -> [w1273]
              tunnel: [w1272] -> w1241
              tunnel: w1242 -> [w1278]
              tunnel: w1241 -> [w1277]
              frame #0 {
                n417 = call-poly <vilib>:"DAQmx Write.vi"("task/channels in"=w1255, "data"=w1254) -> ("error out"=w1253:errorcluster)  [unwired: 11 in, 2 out]
              }
              frame #1 {
                n418 = property on="Delay time" class="DigNum (strict)"() -> ("Value"=w1258:u32)  [unwired: 2 in, 2 out]
                n419 = Wait (ms)(milliseconds to wait=w1258) -> ()  [unwired: 1 out]
              }
              frame #2 {
                n420 = call-poly <vilib>:"DAQmx Write.vi"("task/channels in"=w1267, "data"=TRUE, "error in"=w1264) -> ("task out"=w1265:refnum<k21>, "error out"=w1263:errorcluster)  [unwired: 10 in, 1 out]
              }
              frame #3 {
                n421 = property on="Exposure time" class="DigNum (strict)"() -> ("Value"=w1268:dbl)  [unwired: 2 in, 2 out]
                n422 = Wait (ms)(milliseconds to wait=w1268) -> ()  [unwired: 1 out]
              }
              frame #4 {
                n423 = call-poly <vilib>:"DAQmx Write.vi"("task/channels in"=w1276, "data"=FALSE, "error in"=w1273) -> ("error out"=w1272:errorcluster)  [unwired: 10 in, 2 out]
              }
              frame #5 {
                n424 = while {
                  tunnel: w1278 -> [w1283]
                  tunnel: w1277 -> [w1282]
                  tunnel: [w1281] -> _
                  stop <- w1280 stop-if-true
                  n425 = call-poly <vilib>:"DAQmx Read.vi"("task/channels in"=w1283, "error in"=w1282) -> ("data"=w1279:bool, "error out"=w1281:errorcluster)  [unwired: 11 in, 1 out]
                  n426 = Not(x=w1279) -> (.not. x?=w1280:bool)
                }
              }
            }
            n427 = Add(x=0, y=w1250) -> (x+y=w1229:i32)
            n428 = Index Array(array=i32[] [1, 2, 0, 1, 2, 0, 1, 2, 0, 0, 1, 2, 3, 4, 0], index=w1229) -> (element=w1225:i32)
            n429 = Index Array(array=i32[] [0, 0, 1, 1, 1, 2, 2, 2, 0, 2, 2, 2, 2, 2, 0], index=w1229) -> (element=w1226:i32)
            n430 = Index Array(array=w1252, index (row)=w1225, index (col)=w1226) -> (element=w1227:dbl)
            n431 = property on="Current voltage" class="DigNum (strict)"("Value"=w1227) -> ()  [unwired: 2 in, 2 out]
          }
          frame "Mirror 3" {
            n432 = Index Array(array=w1298, index (row)=2, index (col)=2) -> (element=w1297:dbl)
            n433 = call-poly <vilib>:"DAQmx Write.vi"("task/channels in"=w1299, "data"=w1297) -> ("error out"=w1284:errorcluster)  [unwired: 11 in, 2 out]
            n434 = flat-sequence {
              tunnel: w1286 -> [w1305]
              tunnel: [w1303] -> w1294
              tunnel: w1284 -> [w1302]
              tunnel: [w1301] -> w1293
              tunnel: w1285 -> [w1300]
              tunnel: [w1300] -> w1292
              tunnel: w1294 -> [w1309]
              tunnel: [w1309] -> w1291
              tunnel: w1293 -> [w1307]
              tunnel: [w1308] -> w1290
              tunnel: w1292 -> [w1308]
              tunnel: [w1307] -> w1289
              tunnel: w1291 -> [w1314]
              tunnel: [w1312] -> w1288
              tunnel: w1290 -> [w1312]
              tunnel: w1289 -> [w1311]
              tunnel: [w1310] -> w1287
              tunnel: w1288 -> [w1317]
              tunnel: w1287 -> [w1316]
              tunnel: [w1315] -> _
              frame #0 {
                n435 = call-poly <vilib>:"DAQmx Write.vi"("task/channels in"=w1305, "data"=TRUE, "error in"=w1302) -> ("task out"=w1303:refnum<k21>, "error out"=w1301:errorcluster)  [unwired: 10 in, 1 out]
              }
              frame #1 {
                n436 = property on="Exposure time" class="DigNum (strict)"() -> ("Value"=w1306:dbl)  [unwired: 2 in, 2 out]
                n437 = Wait (ms)(milliseconds to wait=w1306) -> ()  [unwired: 1 out]
              }
              frame #2 {
                n438 = call-poly <vilib>:"DAQmx Write.vi"("task/channels in"=w1314, "data"=FALSE, "error in"=w1311) -> ("error out"=w1310:errorcluster)  [unwired: 10 in, 2 out]
              }
              frame #3 {
                n439 = while {
                  tunnel: w1317 -> [w1322]
                  tunnel: w1316 -> [w1321]
                  tunnel: [w1320] -> w1315
                  stop <- w1318 stop-if-true
                  n440 = call-poly <vilib>:"DAQmx Read.vi"("task/channels in"=w1322, "error in"=w1321) -> ("data"=w1319:bool, "error out"=w1320:errorcluster)  [unwired: 11 in, 1 out]
                  n441 = Not(x=w1319) -> (.not. x?=w1318:bool)
                }
              }
            }
          }
          frame "Party mode" {
            n442 = flat-sequence {
              tunnel: w1329 -> [w1331]
              tunnel: [w1331] -> w1327
              tunnel: w1323 -> [w1330]
              tunnel: [w1336] -> w1328
              tunnel: w1327 -> [w1336]
              tunnel: w1328 -> [w1338]
              tunnel: [w1338] -> w1326
              tunnel: w1323 -> [w1337]
              tunnel: w1326 -> [w1343]
              tunnel: [w1343] -> w1325
              tunnel: w1325 -> [w1345]
              tunnel: [w1345] -> w1324
              tunnel: w1323 -> [w1344]
              tunnel: [w1350] -> _
              tunnel: w1324 -> [w1350]
              frame #0 {
                n443 = Index Array(array=w1331, index (row)=2, index (col)=0) -> (element=w1332:dbl)
                n444 = call-poly <vilib>:"DAQmx Write.vi"("task/channels in"=w1330, "data"=w1332) -> ()  [unwired: 11 in, 3 out]
              }
              frame #1 {
                n445 = property on="Delay time" class="DigNum (strict)"() -> ("Value"=w1335:u32)  [unwired: 2 in, 2 out]
                n446 = Wait (ms)(milliseconds to wait=w1335) -> ()  [unwired: 1 out]
              }
              frame #2 {
                n447 = Index Array(array=w1338, index (row)=2, index (col)=1) -> (element=w1341:dbl)
                n448 = call-poly <vilib>:"DAQmx Write.vi"("task/channels in"=w1337, "data"=w1341) -> ()  [unwired: 11 in, 3 out]
              }
              frame #3 {
                n449 = property on="Delay time" class="DigNum (strict)"() -> ("Value"=w1342:u32)  [unwired: 2 in, 2 out]
                n450 = Wait (ms)(milliseconds to wait=w1342) -> ()  [unwired: 1 out]
              }
              frame #4 {
                n451 = Index Array(array=w1345, index (row)=2, index (col)=2) -> (element=w1346:dbl)
                n452 = call-poly <vilib>:"DAQmx Write.vi"("task/channels in"=w1344, "data"=w1346) -> ()  [unwired: 11 in, 3 out]
              }
              frame #5 {
                n453 = property on="Delay time" class="DigNum (strict)"() -> ("Value"=w1349:u32)  [unwired: 2 in, 2 out]
                n454 = Wait (ms)(milliseconds to wait=w1349) -> ()  [unwired: 1 out]
              }
            }
          }
          frame "Mirror 2" {
            n455 = Index Array(array=w1363, index (row)=2, index (col)=1) -> (element=w1366:dbl)
            n456 = call-poly <vilib>:"DAQmx Write.vi"("task/channels in"=w1362, "data"=w1366) -> ("error out"=w1358:errorcluster)  [unwired: 11 in, 2 out]
            n457 = flat-sequence {
              tunnel: w1361 -> [w1372]
              tunnel: [w1370] -> w1360
              tunnel: w1358 -> [w1369]
              tunnel: [w1368] -> w1357
              tunnel: w1356 -> [w1367]
              tunnel: [w1367] -> w1353
              tunnel: w1360 -> [w1376]
              tunnel: [w1376] -> w1359
              tunnel: w1357 -> [w1374]
              tunnel: [w1375] -> w1354
              tunnel: w1353 -> [w1375]
              tunnel: [w1374] -> w1352
              tunnel: w1359 -> [w1381]
              tunnel: [w1379] -> w1355
              tunnel: w1354 -> [w1379]
              tunnel: w1352 -> [w1378]
              tunnel: [w1377] -> w1351
              tunnel: w1355 -> [w1384]
              tunnel: w1351 -> [w1383]
              tunnel: [w1382] -> _
              frame #0 {
                n458 = call-poly <vilib>:"DAQmx Write.vi"("task/channels in"=w1372, "data"=TRUE, "error in"=w1369) -> ("task out"=w1370:refnum<k21>, "error out"=w1368:errorcluster)  [unwired: 10 in, 1 out]
              }
              frame #1 {
                n459 = property on="Exposure time" class="DigNum (strict)"() -> ("Value"=w1373:dbl)  [unwired: 2 in, 2 out]
                n460 = Wait (ms)(milliseconds to wait=w1373) -> ()  [unwired: 1 out]
              }
              frame #2 {
                n461 = call-poly <vilib>:"DAQmx Write.vi"("task/channels in"=w1381, "data"=FALSE, "error in"=w1378) -> ("error out"=w1377:errorcluster)  [unwired: 10 in, 2 out]
              }
              frame #3 {
                n462 = while {
                  tunnel: w1384 -> [w1389]
                  tunnel: w1383 -> [w1388]
                  tunnel: [w1387] -> w1382
                  stop <- w1386 stop-if-true
                  n463 = call-poly <vilib>:"DAQmx Read.vi"("task/channels in"=w1389, "error in"=w1388) -> ("data"=w1385:bool, "error out"=w1387:errorcluster)  [unwired: 11 in, 1 out]
                  n464 = Not(x=w1385) -> (.not. x?=w1386:bool)
                }
              }
            }
          }
        }
      }
    }
    "?" <- "Go live"
  }
  n465 = stacked-sequence {
    tunnel: w33 -> [w1392 w1410]
    tunnel: w32 -> [w1391 _]
    tunnel: [_ w1409] -> w31
    tunnel: [_ w1408] -> _
    frame #0 {
      n466 = invoke class="MG17Motor" method="SetVelParams"(reference=w1392, error in=w1391, "lChanID"=0, "fMinVel"=0.0, "fAccn"=20, "fMaxVel"=20) -> (reference out=w1399:refnum<k7>, error out=w1398:errorcluster)  [unwired: 1 in, 5 out]
      n467 = property on="561 power" class="Slide (strict)"() -> ("Value"=w1394:dbl)  [unwired: 2 in, 2 out]
      n468 = Multiply(x=45, y=w1394) -> (x*y=w1395:dbl)
      n469 = Add(x=78, y=w1395) -> (x+y=w1393:dbl)
      n470 = invoke class="MG17Motor" method="SetAbsMovePos"(reference=w1399, error in=w1398, "lChanID"=0, "fAbsPos"=w1393) -> (reference out=w1401:refnum<k7>, error out=w1400:errorcluster)  [unwired: 1 in, 3 out]
      n471 = invoke class="MG17Motor" method="MoveAbsolute"(reference=w1401, error in=w1400, "lChanID"=0, "bWait"=TRUE) -> ()  [unwired: 1 in, 5 out]
    }
    frame #1 {
      n472 = while {
        tunnel: [w1416] -> w1409
        tunnel: w1410 -> [w1413]
        tunnel: [w1412] -> w1408
        stop <- w1411 stop-if-true
        n473 = event shown="[0] Timeout" {
          selector: _ -> [_ _]
          dyn-events: _ -> [_ _]
          timeout: 10 -> [_ _]
          tunnel: w1413 -> [w1417 w1425]
          tunnel: [w1417 w1424] -> w1416
          tunnel: "561 power" -> [_ w1420]
          tunnel: [_ w1427] -> w1412
          event Timeout {
            n474 = event-data() -> ()  [unwired: 1 in, 3 out]
          }
          event "561 power": Mouse Up {
            n475 = event-data() -> ()  [unwired: 1 in, 4 out]
            n476 = Multiply(x=45, y=w1420) -> (x*y=w1421:dbl)
            n477 = Add(x=81 ("561 power offset"), y=w1421) -> (x+y=w1419:dbl)
            n478 = invoke class="MG17Motor" method="SetAbsMovePos"(reference=w1425, "lChanID"=0, "fAbsPos"=w1419) -> (reference out=w1423:refnum<k7>)  [unwired: 2 in, 4 out]
            n479 = invoke class="MG17Motor" method="MoveAbsolute"(reference=w1423, "lChanID"=0, "bWait"=TRUE) -> (reference out=w1424:refnum<k7>, error out=w1427:errorcluster)  [unwired: 2 in, 3 out]
          }
        }
        n480 = property on="stop" class="Bool (strict)"() -> ("Value"=w1411:bool)  [unwired: 2 in, 2 out]
      }
    }
  }
  n481 = while {
    tunnel: w70 -> [w1435]
    tunnel: w71 -> [w1436]
    tunnel: [w1436] -> w60
    tunnel: [w1435] -> w59
    tunnel: w26 -> [w1430]
    tunnel: w25 -> [w1433]
    tunnel: [w1432] -> w38
    tunnel: [w1431] -> w37
    stop <- w1434 stop-if-true
    w1437 = 100
    n482 = event shown="[0] Timeout" {
      selector: _ -> [_ _]
      dyn-events: _ -> [_ _]
      timeout: w1437 -> [_ _]
      tunnel: w1433 -> [_ w1464]
      event Timeout {
        n483 = event-data() -> ()  [unwired: 1 in, 3 out]
      }
      event "405": Value Change {
        n484 = event-data() -> ("NewVal"=w1465:bool)  [unwired: 1 in, 5 out]
        n485 = call-poly <vilib>:"DAQmx Write.vi"("task/channels in"=w1464, "data"=w1465) -> ()  [unwired: 11 in, 3 out]
      }
    }
    n486 = event shown="[0] Timeout" {
      selector: _ -> [_ _]
      dyn-events: _ -> [_ _]
      timeout: w1437 -> [_ _]
      tunnel: w1435 -> [_ w1462]
      event Timeout {
        n487 = event-data() -> ()  [unwired: 1 in, 3 out]
      }
      event "488": Value Change {
        n488 = event-data() -> ("NewVal"=w1463:bool)  [unwired: 1 in, 5 out]
        n489 = call-poly <vilib>:"DAQmx Write.vi"("task/channels in"=w1462, "data"=w1463) -> ()  [unwired: 11 in, 3 out]
      }
    }
    n490 = event shown="[0] Timeout" {
      selector: _ -> [_ _]
      dyn-events: _ -> [_ _]
      timeout: w1437 -> [_ _]
      tunnel: w1436 -> [_ w1460]
      event Timeout {
        n491 = event-data() -> ()  [unwired: 1 in, 3 out]
      }
      event "561": Value Change {
        n492 = event-data() -> ("NewVal"=w1461:bool)  [unwired: 1 in, 5 out]
        n493 = call-poly <vilib>:"DAQmx Write.vi"("task/channels in"=w1460, "data"=w1461) -> ()  [unwired: 11 in, 3 out]
      }
    }
    n494 = event shown="[0] Timeout" {
      selector: _ -> [_ _ _]
      dyn-events: _ -> [_ _ _]
      timeout: w1437 -> [_ _ _]
      tunnel: w1430 -> [w1438 w1441 w1455]
      tunnel: [_ w1440 w1452] -> w1431
      tunnel: [w1438 w1439 w1453] -> w1432
      event Timeout {
        n495 = event-data() -> ()  [unwired: 1 in, 3 out]
      }
      event "647": Value Change {
        n496 = event-data() -> ("NewVal"=w1442:bool)  [unwired: 1 in, 5 out]
        n497 = case shown="True" w1442 {
          tunnel: w1441 -> [w1444 w1449]
          tunnel: [w1445 w1448] -> w1440
          tunnel: [w1443 w1447] -> w1439
          frame False {
            n498 = VISA Write(VISA resource name=w1444, write buffer="la off\r" ("format string")) -> (VISA resource name out=w1443:refnum<visa-resource-name>, error out=w1445:errorcluster)  [unwired: 1 in, 1 out]
          }
          frame True {
            n499 = VISA Write(VISA resource name=w1449, write buffer="la on\r" ("format string")) -> (VISA resource name out=w1447:refnum<visa-resource-name>, error out=w1448:errorcluster)  [unwired: 1 in, 1 out]
          }
        }
      }
      event "647 Power": Mouse Up {
        n500 = event-data() -> ()  [unwired: 1 in, 8 out]
        n501 = To Unsigned Byte Integer(number="647 Power") -> (unsigned 8bit integer=w1459:u8)
        n502 = Number To Decimal String(number=w1459) -> (decimal integer string=w1457:string)  [unwired: 1 in]
        n503 = Concatenate Strings("ch 1 pow ", w1457, "\r") -> (w1454:string)
        n504 = VISA Write(VISA resource name=w1455, write buffer=w1454) -> (VISA resource name out=w1453:refnum<visa-resource-name>, error out=w1452:errorcluster)  [unwired: 1 in, 1 out]
      }
    }
    n505 = property on="stop" class="Bool (strict)"() -> ("Value"=w1434:bool)  [unwired: 2 in, 2 out]
  }
  n506 = invoke class="MG17Motor" method="StopCtrl"(reference=w31) -> ()  [unwired: 2 in, 3 out]
  n507 = call <vilib>:"DAQmx Stop Task.vi"("task/channels in"=w9) -> ("task out"=w8:refnum<k21>)  [unwired: 13 in, 1 out]
  n508 = VISA Close(VISA resource name=w38, error in (no error)=w37) -> (error out=w36:errorcluster)
  n509 = call <vilib>:"DAQmx Clear Task.vi"("task in"=w8) -> ("error out"=w7:errorcluster)  [unwired: 14 in]
  n510 = call <vilib>:"DAQmx Stop Task.vi"("task/channels in"=w69) -> ("task out"=w64:refnum<k21>)  [unwired: 13 in, 1 out]
  n511 = call <vilib>:"DAQmx Stop Task.vi"("task/channels in"=w67) -> ("task out"=w66:refnum<k21>)  [unwired: 13 in, 1 out]
  n512 = call-poly <vilib>:"DAQmx Write.vi"("task/channels in"=w59, "data"=w58) -> ("task out"=w55:refnum<k21>, "error out"=w53:errorcluster)  [unwired: 11 in, 1 out]
  n513 = call-poly <vilib>:"DAQmx Write.vi"("task/channels in"=w60, "data"=w58) -> ("task out"=w54:refnum<k21>, "error out"=w52:errorcluster)  [unwired: 11 in, 1 out]
  n514 = call <vilib>:"DAQmx Stop Task.vi"("task/channels in"=w68) -> ("task out"=w65:refnum<k21>)  [unwired: 13 in, 1 out]
  n515 = call <vilib>:"DAQmx Clear Task.vi"("task in"=w64) -> ("error out"=w21:errorcluster)  [unwired: 14 in]
  n516 = call <vilib>:"DAQmx Clear Task.vi"("task in"=w66) -> ("error out"=w62:errorcluster)  [unwired: 14 in]
  n517 = property on="Go live" class="Bool (strict)"(error in=w21, "Value"=FALSE) -> (error out=w20:errorcluster)  [unwired: 1 in, 1 out]
  n518 = call <vilib>:"DAQmx Clear Task.vi"("task in"=w65) -> ("error out"=w61:errorcluster)  [unwired: 14 in]
  n519 = call <vilib>:"DAQmx Stop Task.vi"("task/channels in"=w55, "error in"=w53) -> ("task out"=w56:refnum<k21>, "error out"=w50:errorcluster)  [unwired: 12 in]
  n520 = call <vilib>:"DAQmx Stop Task.vi"("task/channels in"=w54, "error in"=w52) -> ("task out"=w57:refnum<k21>, "error out"=w51:errorcluster)  [unwired: 12 in]
  n521 = Merge Errors(w62, w61, w20, w7) -> (→"Camera/galvo error":errorcluster)
  n522 = call <vilib>:"DAQmx Clear Task.vi"("task in"=w57, "error in"=w51) -> ("error out"=w48:errorcluster)  [unwired: 13 in]
  n523 = call <vilib>:"DAQmx Clear Task.vi"("task in"=w56, "error in"=w50) -> ("error out"=w49:errorcluster)  [unwired: 13 in]
  n524 = Merge Errors(w48, w49, w36) -> (→"Laser error":errorcluster)
  n525 = VISA Close(VISA resource name=w45) -> ()  [unwired: 1 in, 1 out]
